vi "Audio Test.vi"(11 "Module Config":T9={"Name"="Base Station RF Test", "Parent Q"=refnum, "Is Child?"=FALSE, "Index"=0, "Dirs"={"Root"=path "", "Config"=path "C:/ATE/Config", "Logs"=path "C:/ATE/Logs", "Reports"=path "C:/ATE/Reports", "App Data"=path "C:/ProgramData/MAIN"}, "Simulate"=FALSE, "SimCtrl"=refnum}) -> ()   [LabVIEW 2018]
uses:
  <vilib>/KATE/Module/Module Config.ctl
  <vilib>/KATE/Queues/Q.Element.ctl
  <vilib>/KATE/Module/Module.Working Dirs.ctl
  Common/Utils/Results/Result.Measurement Item.ctl
  Common/Utils/Results/Result.Measurement and Attribute Item Status.ctl
  Common/Utils/Results/Result.Results Table Record.ctl
  Common/Utils/Results/Result XML/TestResult.SW Item.ctl
  <vilib>/KATE/Event Log/Event Notification/Event Log.Log Level.ctl
  TypeDefs/SoundCheck Config.ctl
  <vilib>/Utility/miscctls.llb/LVRectTypeDef.ctl
  <vilib>/KATE/Module/Module.SW Version Info.ctl
  <vilib>/KATE/Module/Window/Window.Task, Action.ctl
  Common/Utils/Functions/FunctDataMgr/FunctDataMgr.lvclass
  <vilib>/KATE/SeqMgr/SeqMgr.Result Info.ctl
  <vilib>/KATE/SeqMgr/SeqMgr.Result State Enum.ctl
  <vilib>/KATE/TCP-IP/Mgr/TCP-IP Mgr.Config.ctl
  Common/Utils/Errors/Error.Error Code List.ctl
  Common/Utils/TestExec/TestExec.WorkingDir.ctl
  Common/Utils/TestExec/TestExec.Test Start Message to Sta.ctl
  <vilib>/KATE/Event Log/Event Notification/Event Log.Notification Type.ctl
  Common/Utils/Results/Result.Attribute.ctl
  Common/Utils/Results/Result.Numeric.ctl
  Common/Utils/Results/Result.Limit Type.ctl
  Common/Utils/TestExec/TestExec.Health State Command.ctl
  <vilib>/Utility/config.llb/Read Key (Path).vi
  <vilib>/Utility/config.llb/Read Key (String).vi
  <vilib>/Utility/config.llb/Write Key (Path).vi
  <vilib>/Utility/config.llb/Write Key (String).vi
  <vilib>/KATE/Config/Stored Controls/Class.SaveCtrls.lvclass
  <vilib>/KATE/Queues/Queue Utils.lvlib
  <vilib>/KATE/Module/Module Utils.lvlib
  <vilib>/KATE/Event Log/Event Log.lvlib
  <vilib>/KATE/Scheduler/Scheduler.lvlib
  <vilib>/KATE/Menu/Menu Utils.lvlib
  <vilib>/KATE/Status/Status Utils.lvlib
  <vilib>/KATE/Event Log/Event Notification/Event Notification.lvclass
  <vilib>/KATE/TCP-IP/TCP-IP.lvlib
  <vilib>/KATE/Files/File Utils.lvlib
  <vilib>/KATE/SeqMgr/SeqMgr.lvlib
  <vilib>/KATE/Config/App Data/Class.AppData.lvclass
  <vilib>/KATE/Time/Time Utils.lvlib
  <vilib>/Utility/config.llb/NI_LVConfig.lvlib
panel:
  in  "Main Tab":enum32{"Operate", "Maint"}(tab)
  out "TE":bool
  out "Simulate Indication":string="Simulating Instruments"
  in  "Control Tab":enum32{"Test Control", "Misc Config"}(tab)
  in  "Parse Mic. Seal Results":bool
  in  "Parse Results":bool
  out "Enumerated":bool
  in  "Audio Seq Name":u16(ring)
  in  "Check UUT Enum Status":bool
  in  "Timeout(s)":dbl=500.0 caption="Time Out(s)" format="%.2f"
  in  "Get Top SN":bool
  in  "Mode":string="Production"
  in  "Run SoundCheck Script":bool
  in  "Archive Results":bool
  in  "Init UUT Folder":bool
  out "Start Time":timestamp
  in  "SN":string="ABC123"
  in  "Clear Errors":bool
  in  "Test Reset":bool
  out "Duration(s)":dbl format="%.2g"
  out "Status":string
  in  "Abort":bool
  in  "Result Data Tab":T1(tab)
  in  "Open Summary Dir":bool
  in  "UUT Dir":path caption="UUT Folder"
  in  "Open UUT Dir":bool
  in  "Open Archive Dir":bool
  in  "Filter":string
  in  "Show Only Failures":bool
  in  "Auto Scroll":bool=TRUE
  out "Results Table":T2[](array[typedef]) caption="Results"
  out "Graph Def File":path
  in  "SoundCheck Config":T3={"SeqDir"=path "C:/MTE/Audio Test/Config/SoundCheck/Sequences", "SoundCheckApp"=path "C:/SoundCheck 16.2-x64/SoundCheck 16.2 (x64).exe", "IP"="localhost", "Port"=4444, "Process Name"="SoundCheck 16.2 (x64)", "DataDir"=path "C:/MTE/Audio Test/Data/SoundCheck", "Window"=enum."Minimized"}
  out "Name Lookup":variant
  out "Name Lookup File":path
  in  "Undock HMD Util":bool
  in  "Undock Servo Util":bool
  out "Audio Utuil Dur(s)":dbl format="%.2f"
  out "AudUtil Running":bool
  in  "Run Audio Check":bool
  out "Audio Util Check":T4 {"Status" items=["LOG", "PASS", "FAIL", "ERROR"]}
  in  "Raw Results Tab":enum32{"Raw Result Data", "Other Data"}(tab)
  out "Measurement Data":T4[](array[typedef]) {"Status" items=["LOG", "PASS", "FAIL", "ERROR"]}
  out "Variables":string[][](array[string])
  out "UUT Properties":string[][](array[string])
  out "SW Items":T6[](array[typedef])
  out "Test Running":bool
  out "Error":errorcluster
  out "Ran to completion":bool
  in  "Both Mics":bool
  in  "Right Mic Cover":bool
  in  "Left Mic Cover":bool
  in  "Config - Reset":bool
  in  "Set Window Bounds":bool
  out "Temp Data Dir":path
  out "Archive Summary Dir":path
  out "Archive Dir":path
  in  "Logging Level":T7
  out "Old Window Bounds":T8={"Left"=2142, "Top"=133, "Right"=3354, "Bottom"=889}
  in  "New Window Bounds":T8={"Left"=212, "Top"=78, "Right"=1444, "Bottom"=899}
  out "Rev":string="v1.0.0"
  out "Error Status":string
  out "Title":string
  in  "Leave Maint":bool
  # "Cleanup:"
  # "Step                          Name                                                      Value                                    Units      LimType       LL           UL            Result          Code                     Description"
  # "Name                   PN                      Version                                        Notes"
  # "Name                                                       Value"
  # "Name                                                       Value"
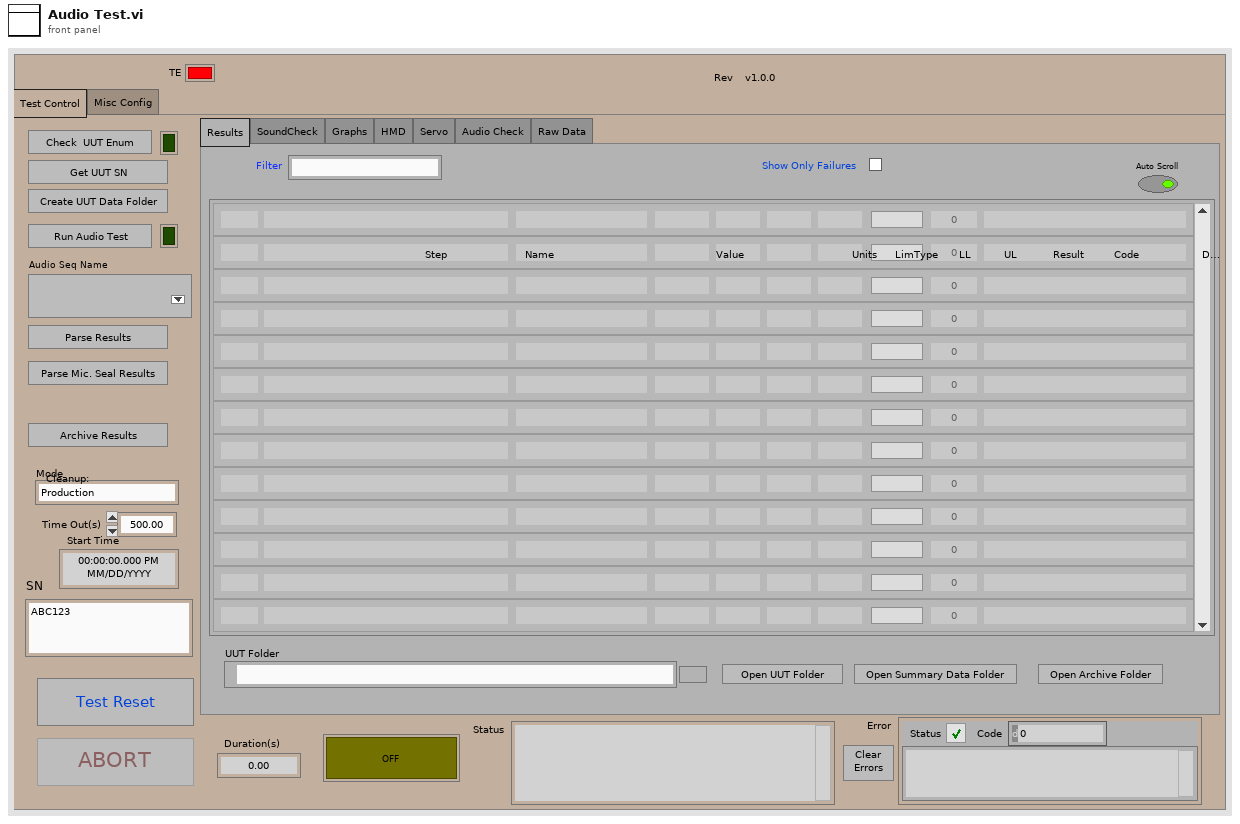
[diagram p1: front panel]
types:
  T1 = enum32{"Results", "SoundCheck", "Graphs", "HMD", "Servo", "Audio Check", "Raw Data"}
  T2 = typedef "Result.Results Table Record.ctl" = cluster{"Cnt":i32, "Step":string, "Category":string, "Name":string, "Value":string, "Units":string, "LimType":string, "LL":string, "UL":string, "Status":string, "Status Color":u32, "Code":i32, "Desc":string}
  T3 = typedef "SoundCheck Config.ctl" = cluster{"SeqDir":path, "SoundCheckApp":path, "IP":string, "Port":u16, "Process Name":string, "DataDir":path, "Window":enum16{"Normal", "Minimized", "Hidden"}}
  T4 = typedef "Result.Measurement Item.ctl" = cluster{"Cnt":i32, "Step":string, "Category":string, "Name":string, "Value":string, "Units":string, "LimType":string, "LL":string, "UL":string, "Status":T5, "Code":i32, "Desc":string, "Time":timestamp}
  T5 = typedef "Result.Measurement and Attribute Item Status.ctl" = i32
  T6 = typedef "TestResult.SW Item.ctl" = cluster{"Name":string, "PN":string, "Version":string, "Note":string}
  T7 = typedef "KATE_Lib.lvlib/Event Log.lvlib/Event Log.Log Level.ctl" = enum16{"Normal", "Verbose", "Debug0", "Debug1", "Debug2"}
  T8 = typedef "LVRectTypeDef.ctl" = cluster{"Left":i16, "Top":i16, "Right":i16, "Bottom":i16}
  T9 = typedef "KATE_Lib.lvlib/Module Utils.lvlib/Module Config.ctl" = cluster{"Name":string, "Parent Q":refnum<queue>, "Is Child?":bool, "Index":i32, "Dirs":T10, "Simulate":bool, "SimCtrl":refnum<vi>}
  T10 = typedef "KATE_Lib.lvlib/Module Utils.lvlib/Module.Working Dirs.ctl" = cluster{"Root":path, "Config":path, "Logs":path, "Reports":path, "App Data":path}
  T11 = typedef "KATE_Lib.lvlib/Module Utils.lvlib/Module.SW Version Info.ctl" = cluster{"AppName":string, "Company":string, "Version":string, "Description":string, "PN":string}
  T12 = typedef "KATE_Lib.lvlib/Module Utils.lvlib/Module Sys Info.ctl" = cluster{"Main Q":refnum<queue>, "Exe":bool, "SW Rev":T11, "Self Ref":refnum<vi>, "Main Tab":refnum<vi>, "Pane":refnum<vi>, "Stop":cluster{"Ref":refnum<event-registration>, "Event":refnum<user-event>}, "Cfg":T9, "Services":cluster{"Name":string, "vi ref":refnum<vi>}[], "Menu Ref":refnum<k9>, "CtrlStates":refnum<class "Class.SaveCtrls.lvclass">, "Docs":cluster{"Tags":string[], "Paths":path[]}, "Log":refnum<class "Event Notification.lvclass">, "Test Controls":refnum<vi>[], "Child Modules":cluster{"Name":string, "vi ref":refnum<vi>}[], "SW Items":string[][], "AppData":refnum<class "Class.AppData.lvclass">, "Subscriptions":refnum<class "Subscription.lvclass">}
  T13 = enum32{"Invalid", "Standard", "Closed", "Hidden", "Minimized", "Maximized"}
  T14 = typedef "KATE_Lib.lvlib/TCP-IP.lvlib/TCP-IP Mgr.Config.ctl" = cluster{"IP":string, "Port":u16, "Listener":bool, "Enable":bool}
  T15 = enum8{"Enabled", "Disabled", "Disabled and Grayed Out"}
  T16 = typedef "KATE_Lib.lvlib/Module Utils.lvlib/Window.Task, Action.ctl" = enum16{"Resize()", "Show Panel(Bool)", "Show Scroll Bars(Bool)", "Dock to SubPanel(SubPanel Ref)", "Undock from SubPanel()", "Return to SubPanel()", "Go To Maint Tab()", "Show Maint Tab(Bool)", "Open Block Diagram()"}
  T17 = typedef "TestExec.WorkingDir.ctl" = cluster{"Name":string, "Path":path}
  T18 = typedef "TestExec.Test Start Message to Sta.ctl" = cluster{"Test Name":string, "Start Time":timestamp, "UUT SN":string}
  T19 = typedef "KATE_Lib.lvlib/Event Log.lvlib/Event Log.Notification Type.ctl" = enum16{"Normal", "Warning", "Error", "Success"}
  T20 = cluster{"State":u16, "Norm":dbl[], "Covered":dbl[]}
  T21 = typedef "Result.Attribute.ctl" = cluster{"Cnt":i32, "Step":string, "Category":string, "Name":string, "Value":string, "Status":T5, "Code":i32, "Desc":string, "Time":timestamp}
  T22 = typedef "Result.Numeric.ctl" = cluster{"Cnt":i32, "Step":string, "Category":string, "Name":string, "Value":dbl, "Units":string, "LimType":T23, "LL":dbl, "UL":dbl, "Status":T5, "Code":i32, "Desc":string, "Time":timestamp}
  T23 = typedef "Result.Limit Type.ctl" = enum16{"None", "EQ", "NE", "GT", "LT", "GE", "LE", "GTLT", "GELE", "GELT", "GTLE", "LTGT", "LEGE", "LEGT", "LTGE", "Contains", "NotContains"}
  T24 = typedef "TestExec.Health State Command.ctl" = enum16{"Update", "Clear All", "Clear Warnings", "Clear Errors", "Set Warning", "Set Error"}
  T25 = typedef "KATE_Lib.lvlib/SeqMgr.lvlib/SeqMgr.Result Info.ctl" = cluster{"State":T26, "Code":i32, "Description":string}
  T26 = typedef "KATE_Lib.lvlib/SeqMgr.lvlib/SeqMgr.Result State Enum.ctl" = enum16{"None", "Passing", "Failing", "PASS", "FAIL", "ABORT", "ERROR"}
  T27 = cluster{"Archive":path, "ArchiveSum":path, "Temp Data":path, "UUTDir":path}
  T28 = cluster{"Lnch":bool, "FunctData":refnum<class "FunctDataMgr.lvclass">, "Timeout(s)":dbl, "Dirs":cluster{"Archive":path, "ArchiveSum":path, "Temp Data":path, "UUTDir":path}, "SN_Time":string, "Remote Test":bool, "ResultState":T25, "StaVer":i32, "Mic":cluster{"State":u16, "Norm":dbl[], "Covered":dbl[]}, "Script":string}
  T29 = typedef "Error.Error Code List.ctl" = i32
  T30 = typedef "NI_LVConfig.lvlib/Config Data RefNum.ctl" = refnum<k1>
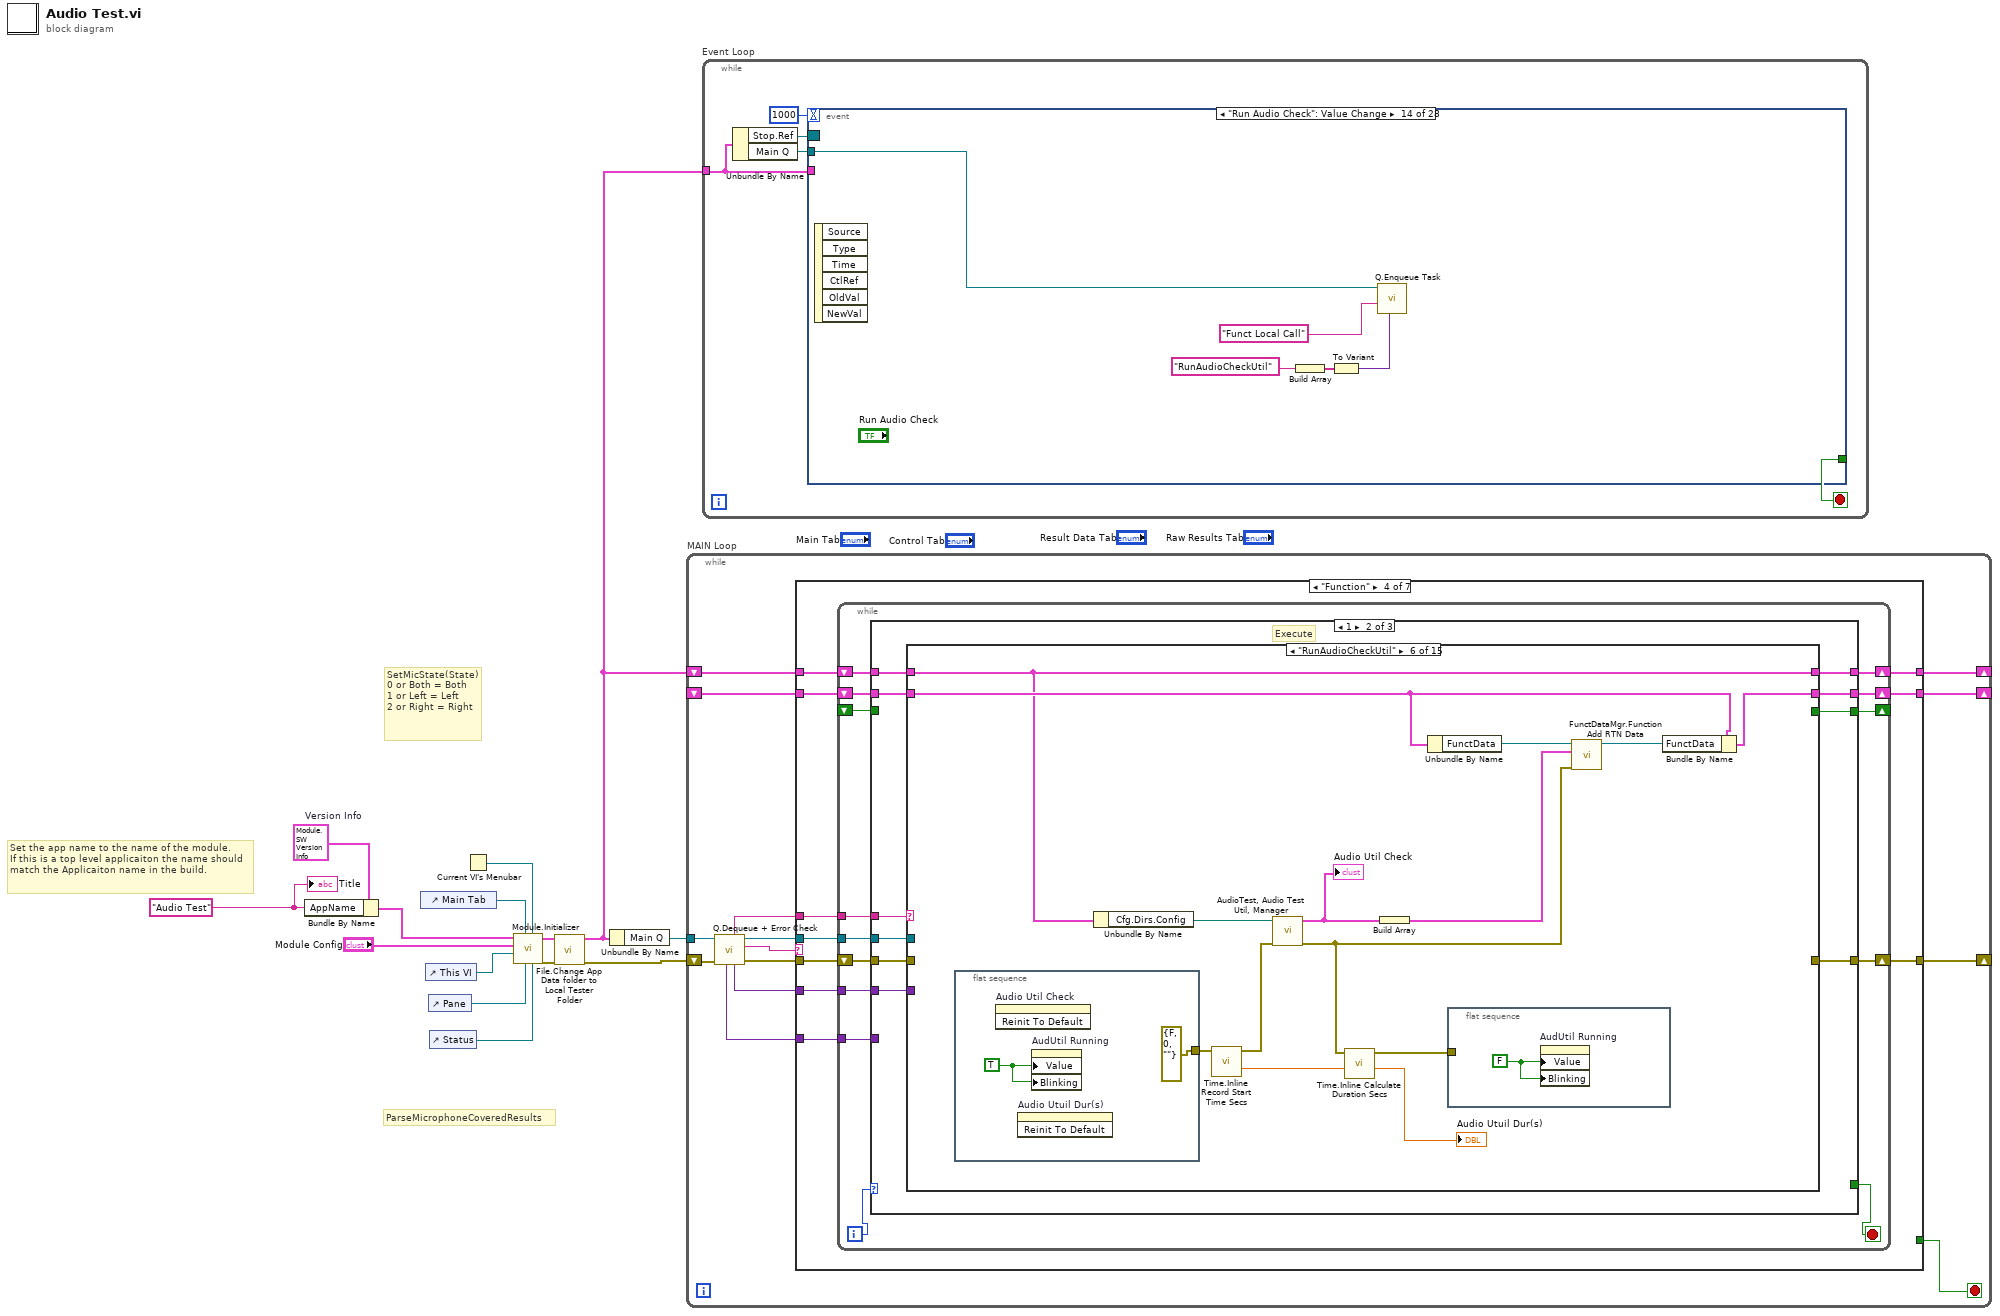
[diagram p0: block diagram]
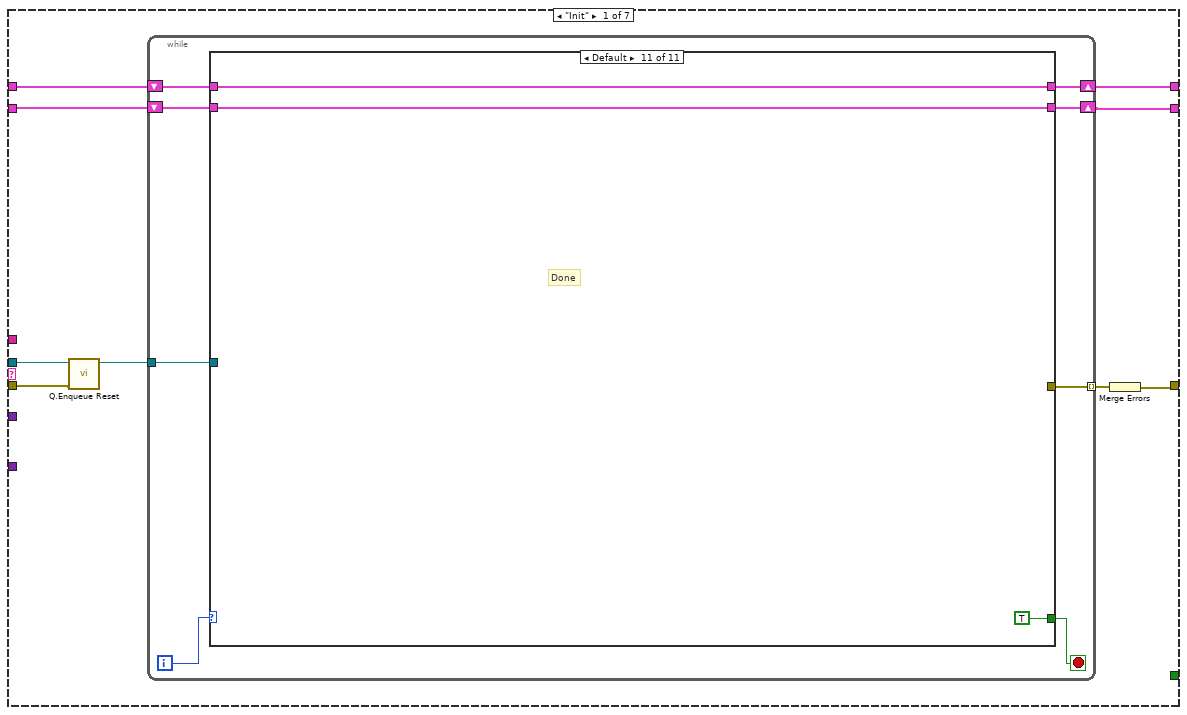
[diagram p2: hidden frame]
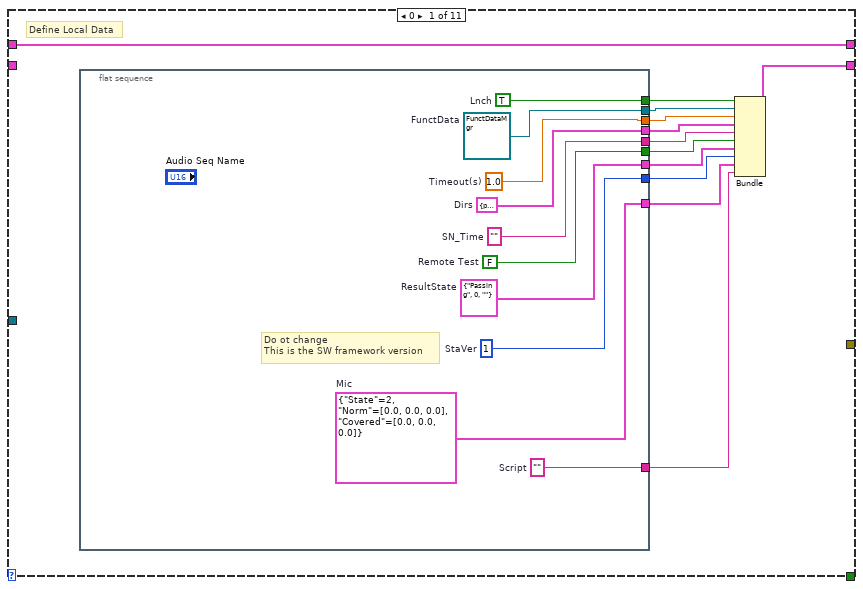
[diagram p3: hidden frame]
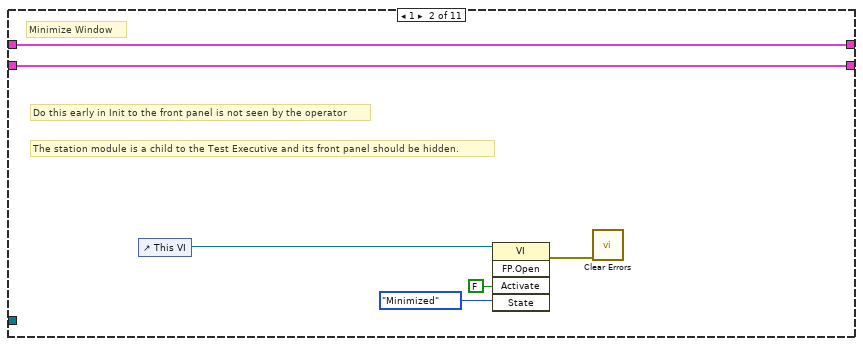
[diagram p4: hidden frame]
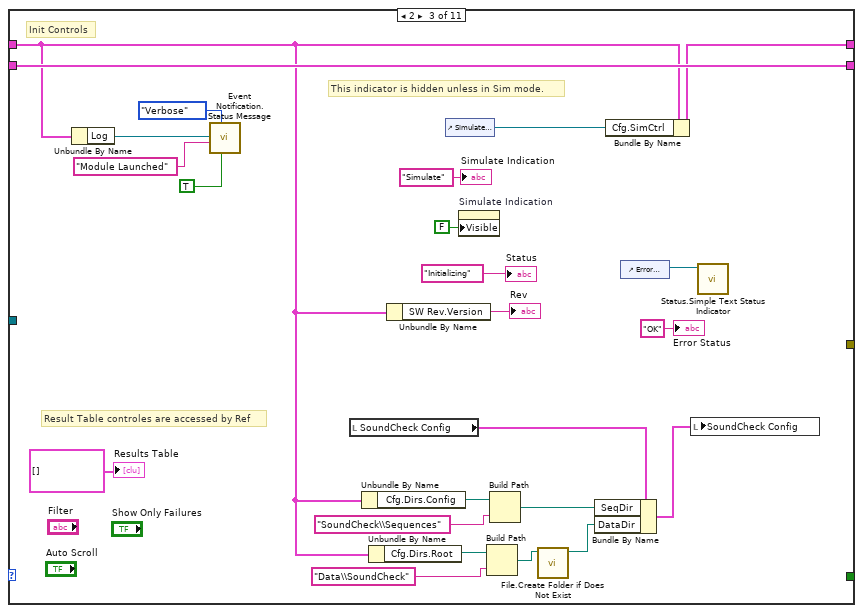
[diagram p5: hidden frame]
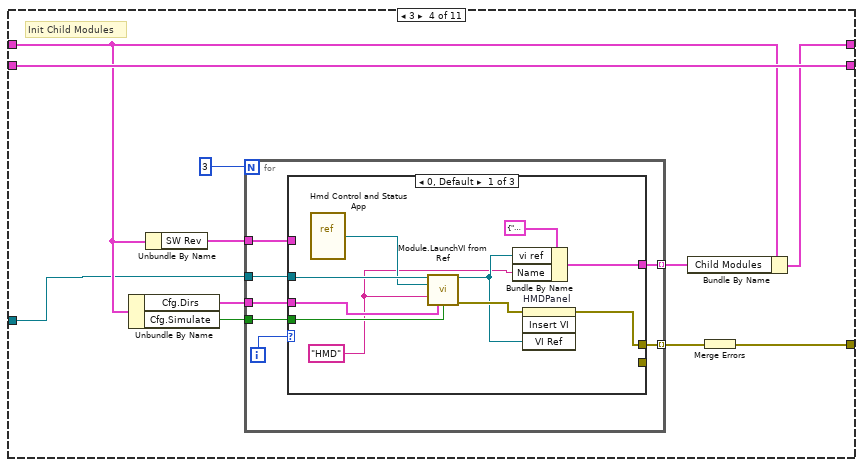
[diagram p6: hidden frame]
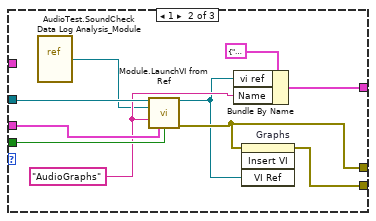
[diagram p7: hidden frame]
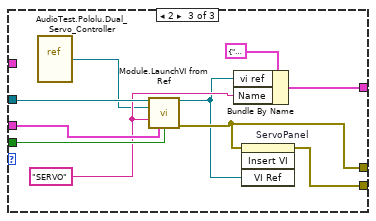
[diagram p8: hidden frame]
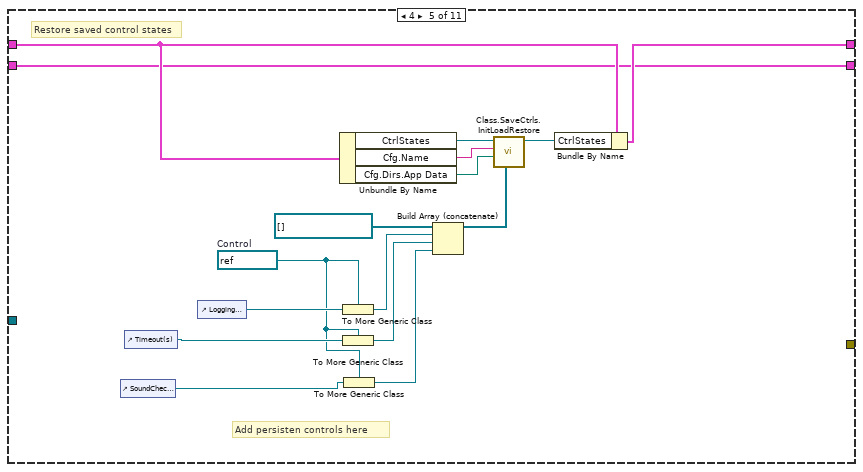
[diagram p9: hidden frame]
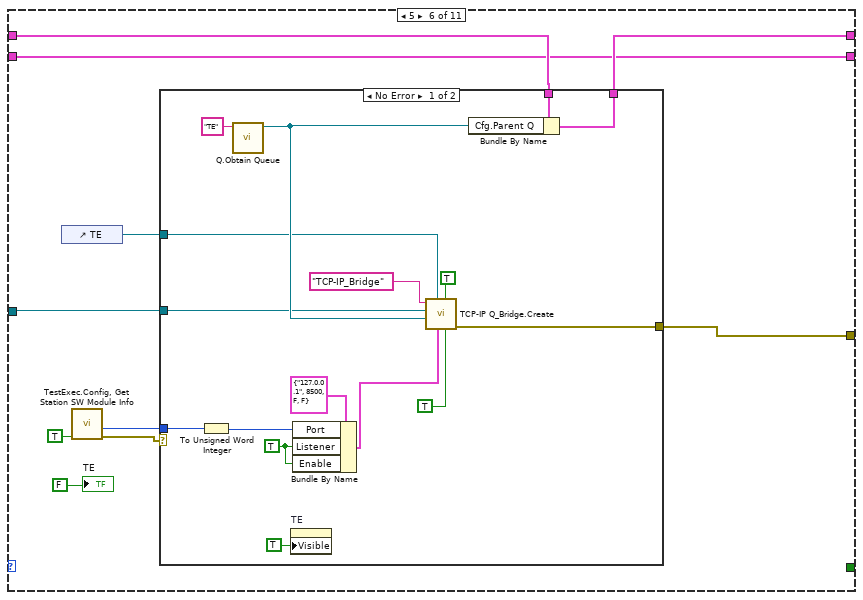
[diagram p10: hidden frame]
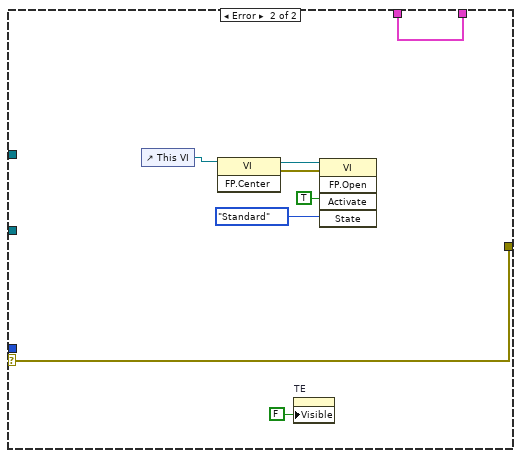
[diagram p11: hidden frame]
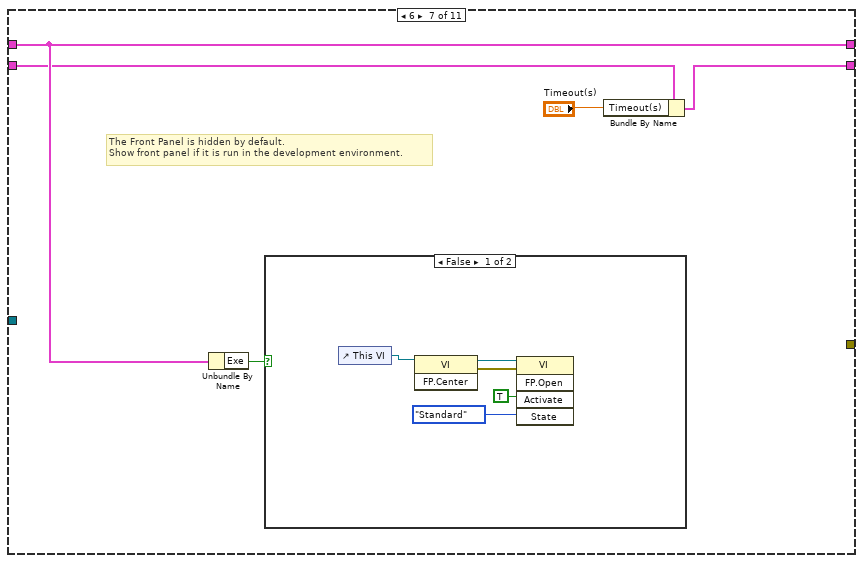
[diagram p12: hidden frame]
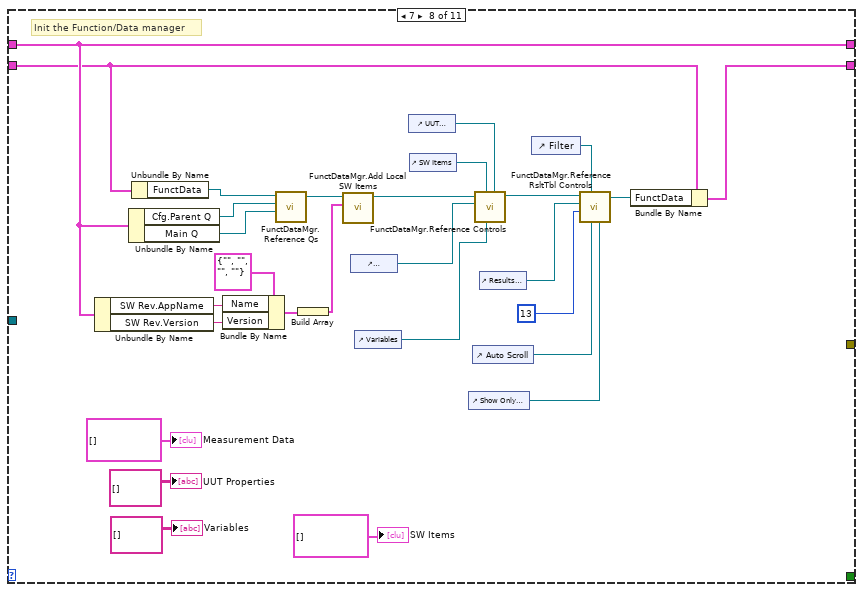
[diagram p14: hidden frame]
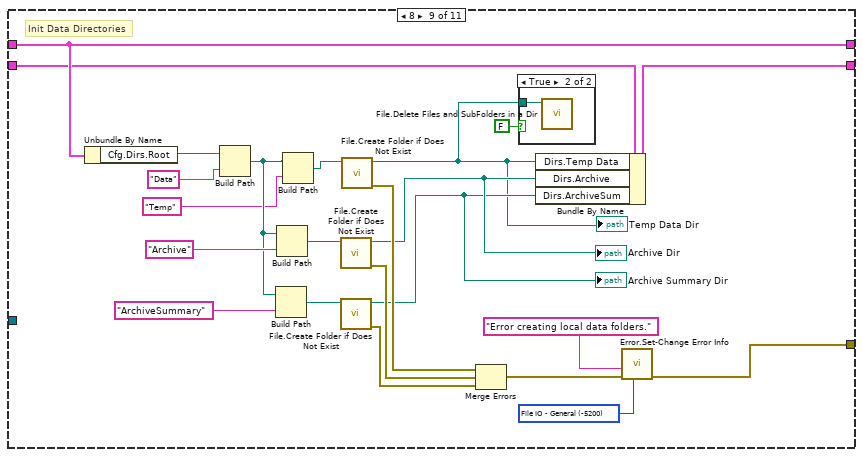
[diagram p15: hidden frame]
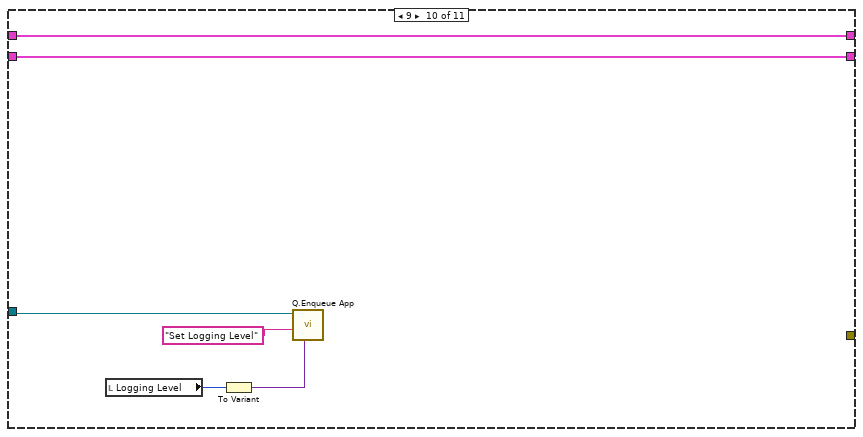
[diagram p17: hidden frame]
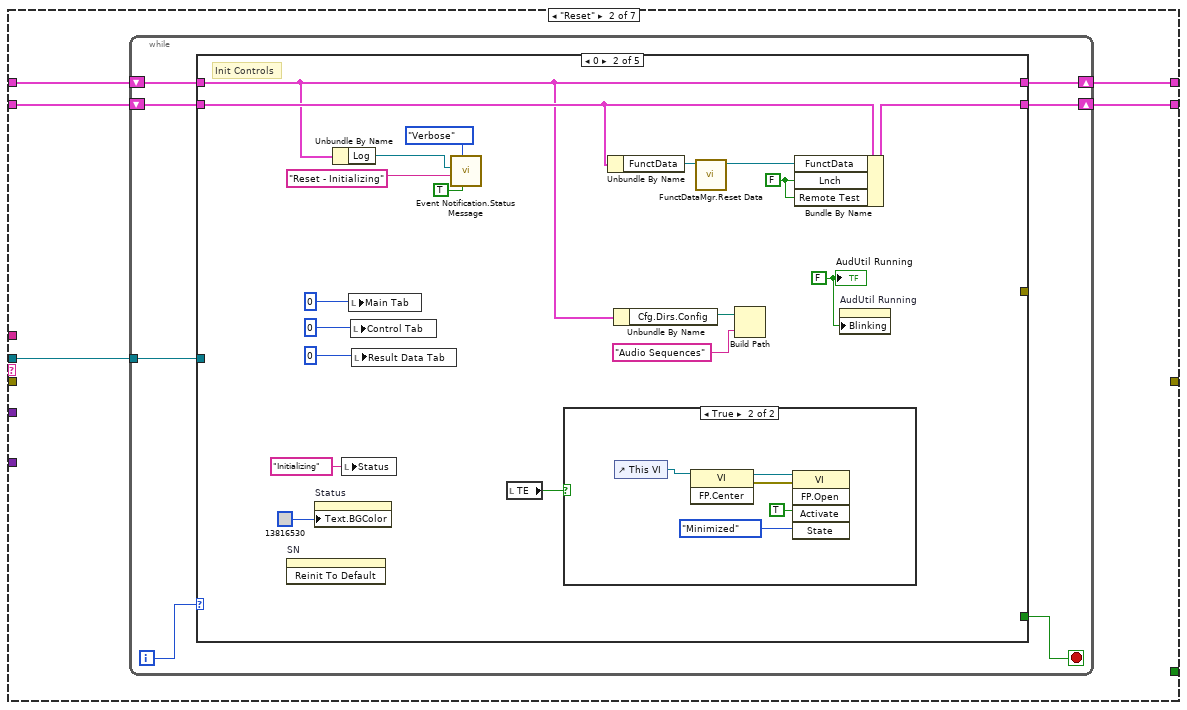
[diagram p18: hidden frame]
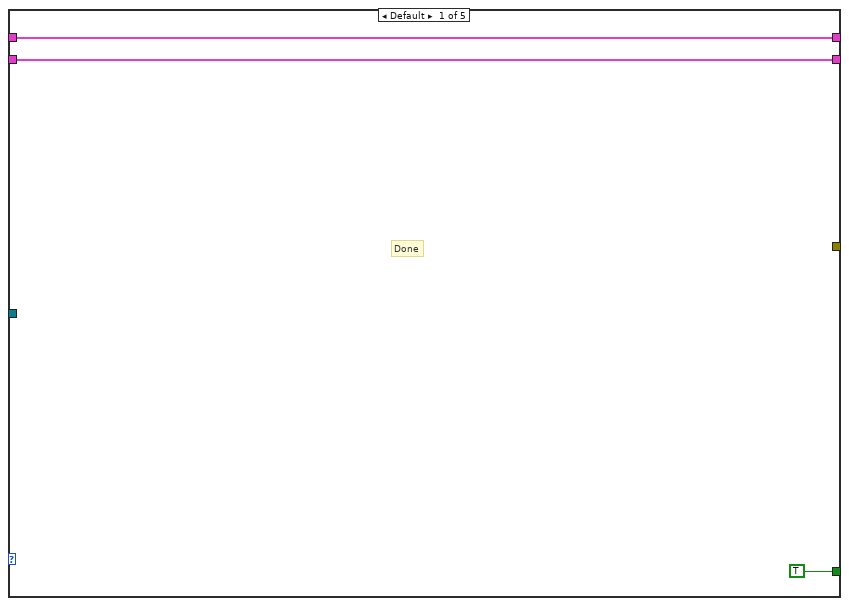
[diagram p19: hidden frame]
diagram:
  w8 = T11 {"AppName"="ModuleX", "Company"="CompanyX", "Version"="1.0", "Description"="This app is being developed.", "PN"=""}  # Version Info
  w5 = "Audio Test"
  # "ParseMicrophoneCoveredResults"
  # "SetMicState(State)\n0 or Both = Both\n1 or Left = Left\n2 or Right = Right"
  # "Set the app name to the name of the module.\nIf this is a top level applicaiton the name should match the Applicaiton name in the build."
  n1 = Bundle By Name(cluster=w8, "AppName"=w5) -> (w7:T11)
  n2 = control-ref of="Main Tab"() -> (w13:refnum<vi>)
  n3 = control-ref of="This VI"() -> (w12:refnum<vi>)
  n4 = control-ref of="Pane"() -> (w11:refnum<vi>)
  n5 = control-ref of="Status"() -> (w6:refnum<vi>)
  n6 = Current VI's Menubar() -> (w10:refnum<k9>)
  n7 = call <vilib>:"Module.Initializer.vi"("StatusTxtBx"=w6, "Menu Ref"=w10, "Pane"=w11, "Main Tab"=w13, "Self Ref"=w12, "Module Config"="Module Config", "SW Rev"=w7) -> ("error out"=w3:errorcluster, "Sys"=w2:T12)  [unwired: 3 in]
  n8 = call "File.Change App Data folder to Local Tester Folder.vi"("Sys"=w2) -> ("Sys Out"=w1:T12)  [unwired: 9 in, 1 out]
  n9 = Unbundle By Name(w1) -> ("Main Q"=w4:refnum<queue>)
  n10 = while "MAIN Loop" {
    shift-right: [w23] -> _
    shift-left: w3 -> [w21]
    shift-right: [w24] -> _
    shift-left: _ -> [w27]
    shift-right: [w25] -> _
    shift-left: w1 -> [w26]
    tunnel: w4 -> [w20]
    stop <- w16 stop-if-true
    n11 = call <vilib>:"Q.Dequeue + Error Check.vi"("Error In"=w21, "Q In"=w20) -> ("error out"=w22:errorcluster, "Cmd"=w15:string, "Q Out"=w19:refnum<queue>, "Data1"=w18:variant, "Sub"=w14:string, "Data2"=w17:variant)  [unwired: 4 in]
    n12 = case shown="\"Function\"" w15 {
      selector: w15 -> [_ _ _ _ _ w1245 _]
      tunnel: w27 -> [w32 w269 w368 w838 w1194 w1251 w1298]
      tunnel: w26 -> [w34 w270 w369 w839 w1195 w1250 w1294]
      tunnel: [w33 w268 w367 w837 w1193 w1250 w1295] -> w25
      tunnel: [w31 w267 w366 w836 w1192 w1249 w1298] -> w24
      tunnel: [w28 _ w360 w834 _ w1248 w1300] -> w23
      tunnel: w22 -> [w35 _ w362 w835 _ w1244 _]
      tunnel: w19 -> [w36 w266 w363 w832 w1198 w1247 _]
      tunnel: w18 -> [_ _ w364 w831 w1197 w1243 _]
      tunnel: w17 -> [_ _ w361 w830 w1196 _ _]
      tunnel: w14 -> [_ _ w365 w833 w1199 w1246 _]
      tunnel: [_ _ _ _ _ _ TRUE] -> w16
      frame "Init" {
        n13 = call <vilib>:"Q.Enqueue Reset.vi"("Error In"=w35, "Q In"=w36) -> ("Q Out"=w30:refnum<queue>)  [unwired: 8 in, 1 out]
        n14 = while {
          shift-right: [w43] -> w33
          shift-left: w34 -> [w44]
          shift-right: [w41] -> w31
          shift-left: w32 -> [w42]
          tunnel: w30 -> [w39]
          tunnel: [w38] -> w29 mode=indexing
          i -> [w37]
          stop <- w40 stop-if-true
          n15 = case shown="Default" w37 {
            tunnel: w44 -> [w56 w72 w77 w99 w151 w164 w198 w214 w255 w262 w265]
            tunnel: [w56 w72 w87 w100 w149 w163 w198 w214 w255 w262 w265] -> w43
            tunnel: w42 -> [_ w69 w96 w107 w148 w162 w197 w211 w254 w261 w264]
            tunnel: [w55 w69 w96 w107 w148 w162 w196 w212 w253 w261 w264] -> w41
            tunnel: [_ _ _ _ _ _ _ _ _ _ TRUE] -> w40
            tunnel: w39 -> [_ _ _ w98 _ w165 _ _ _ w258 _]
            tunnel: [_ _ _ w101 _ w161 _ _ w243 _ _] -> w38
            frame 0 {
              # "Define Local Data"
              n16 = flat-sequence {
                tunnel: [w66] -> w54
                tunnel: [w65] -> w53
                tunnel: [w64] -> w52
                tunnel: [w63] -> w51
                tunnel: [w62] -> w50
                tunnel: [w61] -> w49
                tunnel: [w60] -> w48
                tunnel: [w59] -> w47
                tunnel: [w58] -> w46
                tunnel: [w57] -> w45
                frame #0 {
                  w57 = ""  # Script
                  w58 = T20 {"State"=2, "Norm"=[0.0, 0.0, 0.0], "Covered"=[0.0, 0.0, 0.0]}  # Mic
                  w59 = 1  # StaVer
                  w60 = T25 {"State"=enum."Passing", "Code"=0, "Description"=""}  # ResultState
                  w61 = FALSE  # Remote Test
                  w62 = ""  # SN_Time
                  w65 = refnum<class "FunctDataMgr.lvclass"> refnum  # FunctData
                  w63 = T27 {"Archive"=path "", "ArchiveSum"=path "", "Temp Data"=path "", "UUTDir"=path ""}  # Dirs
                  w64 = 1.0  # Timeout(s)
                  w66 = TRUE  # Lnch
                  # "Do ot change\nThis is the SW framework version"
                }
              }
              n17 = Bundle("Lnch"=w54, "FunctData"=w53, "Timeout(s)"=w52, "Dirs"=w51, "SN_Time"=w50, "Remote Test"=w49, "ResultState"=w48, "StaVer"=w47, "Mic"=w46, "Script"=w45) -> (w55:T28)  [unwired: 1 in]
            }
            frame 1 {
              # "The station module is a child to the Test Executive and its front panel should be hidden."
              # "Do this early in Init to the front panel is not seen by the operator"
              # "Minimize Window"
              n18 = control-ref of="This VI"() -> (w68:refnum<vi>)
              n19 = invoke class="VI" method="FP.Open"(reference=w68, "Activate"=FALSE ("Activate?"), "State"=T13."Minimized") -> (error out=w67:errorcluster)  [unwired: 2 in, 4 out]
              n20 = call <vilib>:"Clear Errors.vi"("error in (no error)"=w67) -> ()  [unwired: 5 in, 2 out]
            }
            frame 2 {
              # "Init Controls"
              # "This indicator is hidden unless in Sim mode."
              # "Result Table controles are accessed by Ref"
              n21 = Unbundle By Name(w77) -> ("Log"=w94:refnum<class "Event Notification.lvclass">)
              n22 = call <vilib>:"Event Notification.Status Message.vi"("Log"=TRUE, "Level"=Event_Log.Log_Level."Verbose", "Message"="Module Launched", "Event Notification in"=w94) -> ()  [unwired: 8 in]
              n23 = local read "SoundCheck Config"() -> (w82:T3)
              n24 = Unbundle By Name(w77) -> ("Cfg.Dirs.Config"=w80:path)
              n25 = Unbundle By Name(w77) -> ("Cfg.Dirs.Root"=w76:path)
              n26 = Unbundle By Name(w77) -> ("SW Rev.Version"=→"Rev":string)
              n27 = control-ref of="Simulate Indication"() -> (w88:refnum<vi>)
              n28 = property on="Simulate Indication" class="Str"("Visible"=FALSE) -> ()  [unwired: 2 in, 2 out]
              n29 = Build Path(base path=w76, name or relative path="Data\\SoundCheck") -> (appended path=w73:path)
              n30 = Build Path(base path=w80, name or relative path="SoundCheck\\Sequences") -> (appended path=w78:path)
              n31 = call <vilib>:"File.Create Folder if Does Not Exist.vi"("Path"=w73) -> ("Dup Path"=w74:path)  [unwired: 8 in, 2 out]
              n32 = Bundle By Name(cluster=w82, "SeqDir"=w78, "DataDir"=w74) -> (w81:T3)
              n33 = Bundle By Name(cluster=w77, "Cfg.SimCtrl"=w88) -> (w87:T12)
              n34 = control-ref of="Error Status"() -> (w86:refnum<vi>)
              n35 = local write "SoundCheck Config"(w81) -> ()
              n36 = call <vilib>:"Status.Simple Text Status Indicator.vi"("Status TextBox"=w86) -> ()  [unwired: 10 in, 1 out]
              "Results Table" <- T2[] [] ("Results Table")
              "Simulate Indication" <- "Simulate" ("Simulate Indication")
              "Status" <- "Initializing" ("Status")
              "Error Status" <- "OK" ("Error Status")
            }
            frame 3 {
              # "Init Child Modules"
              n37 = Unbundle By Name(w99) -> ("Cfg.Dirs"=w104:T10, "Cfg.Simulate"=w105:bool)
              n38 = Unbundle By Name(w99) -> ("SW Rev"=w103:T11)
              n39 = for {
                N: 3 -> [_]
                tunnel: w103 -> [w114]
                tunnel: [w109] -> w97 mode=indexing
                tunnel: w98 -> [w112]
                tunnel: w104 -> [w111]
                tunnel: w105 -> [w110]
                tunnel: [w108] -> w106 mode=indexing
                i -> [w113]
                n40 = case shown="0, Default" w113 {
                  tunnel: w114 -> [_ _ _]
                  tunnel: w112 -> [w124 w134 w144]
                  tunnel: w111 -> [w118 w132 w142]
                  tunnel: w110 -> [w117 w131 w141]
                  tunnel: [w122 w133 w143] -> w109
                  tunnel: [w121 w128 w138] -> w108
                  tunnel: [_ w127 w137] -> _
                  frame 0, Default {
                    w115 = "HMD"
                    n41 = vi-ref "Hmd Control and Status App.vi"() -> (w123:refnum<vi>)
                    n42 = call <vilib>:"Module.LaunchVI from Ref.vi"("Parent Q"=w124, "VI Ref In"=w123, "Q Name"=w115, "Working Dirs"=w118, "Simulate"=w117) -> ("VI Ref Out"=w119:refnum<vi>, "error out"=w120:errorcluster)  [unwired: 8 in, 1 out]
                    n43 = Bundle By Name(cluster=cluster{"Name":string, "vi ref":refnum<vi>} {"Name"="", "vi ref"=refnum} ("Service"), "vi ref"=w119, "Name"=w115) -> (w122:cluster{"Name":string, "vi ref":refnum<vi>})
                    n44 = invoke on="HMDPanel" class="SubPnl" method="Insert VI"(error in=w120, "VI Ref"=w119) -> (error out=w121:errorcluster)  [unwired: 2 in, 3 out]
                  }
                  frame 1 {
                    w129 = "AudioGraphs"
                    n45 = vi-ref "AudioTest.SoundCheck Data Log Analysis_Module.vi"() -> (w125:refnum<vi>)
                    n46 = call <vilib>:"Module.LaunchVI from Ref.vi"("Parent Q"=w134, "VI Ref In"=w125, "Q Name"=w129, "Working Dirs"=w132, "Simulate"=w131) -> ("VI Ref Out"=w126:refnum<vi>, "error out"=w128:errorcluster)  [unwired: 8 in, 1 out]
                    n47 = Bundle By Name(cluster=cluster{"Name":string, "vi ref":refnum<vi>} {"Name"="", "vi ref"=refnum} ("Service"), "vi ref"=w126, "Name"=w129) -> (w133:cluster{"Name":string, "vi ref":refnum<vi>})
                    n48 = invoke on="Graphs" class="SubPnl" method="Insert VI"(error in=w128, "VI Ref"=w126) -> (error out=w127:errorcluster)  [unwired: 2 in, 3 out]
                  }
                  frame 2 {
                    w139 = "SERVO"
                    n49 = vi-ref "AudioTest.Pololu.Dual_Servo_Controller.vi"() -> (w135:refnum<vi>)
                    n50 = call <vilib>:"Module.LaunchVI from Ref.vi"("Parent Q"=w144, "VI Ref In"=w135, "Q Name"=w139, "Working Dirs"=w142, "Simulate"=w141) -> ("VI Ref Out"=w136:refnum<vi>, "error out"=w138:errorcluster)  [unwired: 8 in, 1 out]
                    n51 = Bundle By Name(cluster=cluster{"Name":string, "vi ref":refnum<vi>} {"Name"="", "vi ref"=refnum} ("Service"), "vi ref"=w136, "Name"=w139) -> (w143:cluster{"Name":string, "vi ref":refnum<vi>})
                    n52 = invoke on="ServoPanel" class="SubPnl" method="Insert VI"(error in=w138, "VI Ref"=w136) -> (error out=w137:errorcluster)  [unwired: 2 in, 3 out]
                  }
                }
              }
              n53 = Bundle By Name(cluster=w99, "Child Modules"=w97) -> (w100:T12)
              n54 = Merge Errors(w106) -> (w101:errorcluster)
            }
            frame 4 {
              w146 = refnum<vi> refnum  # Control
              # "Add persisten controls here"
              # "Restore saved control states"
              n55 = control-ref of="SoundCheck Config"() -> (w147:refnum<vi>)
              n56 = control-ref of="Timeout(s)"() -> (w150:refnum<vi>)
              n57 = control-ref of="Logging Level"() -> (w160:refnum<vi>)
              n58 = Unbundle By Name(w151) -> ("CtrlStates"=w156:refnum<class "Class.SaveCtrls.lvclass">, "Cfg.Name"=w154:string, "Cfg.Dirs.App Data"=w155:path)
              n59 = To More Generic Class(target class=w146, reference=w160) -> (generic class reference=w158:refnum<vi>)
              n60 = To More Generic Class(target class=w146, reference=w150) -> (generic class reference=w159:refnum<vi>)
              n61 = To More Generic Class(target class=w146, reference=w147) -> (generic class reference=w145:refnum<vi>)
              n62 = Build Array (concatenate)(refnum<vi>[] [], w158, w159, w145) -> (w157:refnum<vi>[])
              n63 = call-dynamic "Class.SaveCtrls.InitLoadRestore.vi"("Ctrl Array"=w157, "Module Data Dir"=w155, "Module Name"=w154, "CtrlStates In"=w156) -> ("CtrlStates"=w152:refnum<class "Class.SaveCtrls.lvclass">)  [unwired: 6 in, 1 out]
              n64 = Bundle By Name(cluster=w151, "CtrlStates"=w152) -> (w149:T12)
            }
            frame 5 {
              n65 = control-ref of="TE"() -> (w170:refnum<vi>)
              n66 = call "TestExec.Config, Get Station SW Module Info.vi"("Error if File Doesn't Exist"=TRUE) -> ("error out"=w169:errorcluster, "Station IP Port"=w168:i32)  [unwired: 7 in, 2 out]
              n67 = case shown="No Error" w169 {
                selector: w169 -> [_ w193]
                tunnel: w164 -> [w186 w194]
                tunnel: [w185 w194] -> w163
                tunnel: w168 -> [w178 _]
                tunnel: w165 -> [w175 _]
                tunnel: [w174 w193] -> w161
                tunnel: w170 -> [w173 _]
                frame No Error {
                  w179 = TRUE ("Listener")
                  n68 = To Unsigned Word Integer(number=w178) -> (unsigned 16bit integer=w177:u16)
                  n69 = call <vilib>:"Q.Obtain Queue.vi"("Q Name"="TE") -> ("Q Out"=w183:refnum<queue>)  [unwired: 8 in, 2 out]
                  n70 = property on="TE" class="Bool (strict)"("Visible"=TRUE) -> ()  [unwired: 2 in, 2 out]
                  n71 = Bundle By Name(cluster=T14 {"IP"="127.0.0.1", "Port"=8500, "Listener"=FALSE, "Enable"=FALSE} ("Config"), "Port"=w177, "Listener"=w179, "Enable"=w179) -> (w180:T14)
                  n72 = call <vilib>:"TCP-IP Q_Bridge.Create.vi"("Auto Exit"=TRUE, "Notification"=TRUE, "Config"=w180, "StatusCtrlRef"=w173, "Q_DataOut"=w183, "Q_DataIn"=w175, "Control Q Name"="TCP-IP_Bridge" ("Control Q")) -> ("Error Out"=w174:errorcluster)  [unwired: 3 in, 1 out]
                  n73 = Bundle By Name(cluster=w186, "Cfg.Parent Q"=w183) -> (w185:T12)
                }
                frame Error {
                  n74 = control-ref of="This VI"() -> (w189:refnum<vi>)
                  n75 = invoke class="VI" method="FP.Center"(reference=w189) -> (reference out=w190:refnum<vi>, error out=w191:errorcluster)  [unwired: 2 in, 1 out]
                  n76 = property on="TE" class="Bool (strict)"("Visible"=FALSE) -> ()  [unwired: 2 in, 2 out]
                  n77 = invoke class="VI" method="FP.Open"(reference=w190, error in=w191, "Activate"=TRUE ("Activate?"), "State"=T13."Standard") -> ()  [unwired: 1 in, 5 out]
                }
              }
              "TE" <- FALSE ("Sta")
            }
            frame 6 {
              # "The Front Panel is hidden by default.\nShow front panel if it is run in the development environment."
              n78 = Unbundle By Name(w198) -> ("Exe"=w199:bool)
              n79 = case shown="False" w199 {
                frame False {
                  n80 = control-ref of="This VI"() -> (w202:refnum<vi>)
                  n81 = invoke class="VI" method="FP.Center"(reference=w202) -> (reference out=w203:refnum<vi>, error out=w204:errorcluster)  [unwired: 2 in, 1 out]
                  n82 = invoke class="VI" method="FP.Open"(reference=w203, error in=w204, "Activate"=TRUE ("Activate?"), "State"=T13."Standard") -> ()  [unwired: 1 in, 5 out]
                }
                frame True {
                }
              }
              n83 = Bundle By Name(cluster=w197, "Timeout(s)"="Timeout(s)") -> (w196:T28)
            }
            frame 7 {
              # "Init the Function/Data manager"
              n84 = Unbundle By Name(w214) -> ("SW Rev.AppName"=w219:string, "SW Rev.Version"=w220:string)
              n85 = Unbundle By Name(w214) -> ("Cfg.Parent Q"=w222:refnum<queue>, "Main Q"=w223:refnum<queue>)
              n86 = Unbundle By Name(w211) -> ("FunctData"=w210:refnum<class "FunctDataMgr.lvclass">)
              n87 = Bundle By Name(cluster=T6 {"Name"="", "PN"="", "Version"="", "Note"=""} ("SW"), "Name"=w219, "Version"=w220) -> (w218:T6)
              n88 = call "FunctDataMgr.Reference Qs.vi"("Q Local"=w223, "Q Parent"=w222, "FunctDataMgr in"=w210) -> ("FunctDataMgr"=w224:refnum<class "FunctDataMgr.lvclass">)  [unwired: 7 in, 1 out]
              n89 = Build Array(w218) -> (w221:T6[])
              n90 = call "FunctDataMgr.Add Local SW Items.vi"("Local SW Items"=w221, "FunctDataMgr in"=w224) -> ("FunctDataMgr"=w225:refnum<class "FunctDataMgr.lvclass">)  [unwired: 8 in, 1 out]
              n91 = control-ref of="Measurement Data"() -> (w205:refnum<vi>)
              n92 = control-ref of="Variables"() -> (w232:refnum<vi>)
              n93 = control-ref of="UUT Properties"() -> (w226:refnum<vi>)
              n94 = control-ref of="SW Items"() -> (w227:refnum<vi>)
              n95 = control-ref of="Show Only Failures"() -> (w230:refnum<vi>)
              n96 = control-ref of="Auto Scroll"() -> (w231:refnum<vi>)
              n97 = call "FunctDataMgr.Reference Controls.vi"("UUTProps"=w226, "Vars"=w232, "SWItems"=w227, "Ctrls.MeasData"=w205, "FunctDataMgr in"=w225) -> ("FunctDataMgr"=w217:refnum<class "FunctDataMgr.lvclass">)  [unwired: 5 in, 1 out]
              n98 = control-ref of="Results Table"() -> (w229:refnum<vi>)
              n99 = control-ref of="Filter"() -> (w228:refnum<vi>)
              n100 = call "FunctDataMgr.Reference RsltTbl Controls.vi"("ShowOnlyFail"=w230, "AutoScroll"=w231, "Filter"=w228, "Visible Rows"=13, "RsltTbl"=w229, "FunctDataMgr in"=w217) -> ("FunctDataMgr"=w213:refnum<class "FunctDataMgr.lvclass">)  [unwired: 4 in, 1 out]
              n101 = Bundle By Name(cluster=w211, "FunctData"=w213) -> (w212:T28)
              "Measurement Data" <- T4[] [] ("Numeric Data")
              "UUT Properties" <- string[][] [] ("UUT Properties")
              "Variables" <- string[][] [] ("Variables")
              "SW Items" <- T6[] [] ("SW Items")
            }
            frame 8 {
              w242 = T29 -5200 items=["No Error"=0, "Abort"=-2, "Misc"=-5000, "Fixture Error"=-5100, "File IO - General"=-5200, "FIle IO - Config Error"=-5201, "Instrument - General"=-5300, "Instrument - Serial Com"=-5301, "Instrument - Camera"=-5302, "Instrument - PS"=-5303, "Instrument - Oscilloscope"=-5304, "Instrument - Function Gen"=-5305, "Instrument - Load"=-5306, "Instrument - Meter"=-5307, "Instrument - Power Control"=-5308, "Instrument - Motion"=-5309, "Instrument - RF"=-5310, "System Exe"=-5400, "Image Processing"=-5500, "Communication"=-5600, "Script - Syntax Error"=-6000, "Script - Invalid Name or Param"=-6100, "Script - Timeout"=-6200, "Invalid Data"=-6300, "FW Update Error"=-6500] ("Std Code")
              # "Init Data Directories"
              n102 = Unbundle By Name(w255) -> ("Cfg.Dirs.Root"=w252:path)
              n103 = Build Path(base path=w252, name or relative path="Data") -> (appended path=w240:path)
              n104 = Build Path(base path=w240, name or relative path="ArchiveSummary") -> (appended path=w237:path)
              n105 = Build Path(base path=w240, name or relative path="Archive") -> (appended path=w250:path)
              n106 = Build Path(base path=w240, name or relative path="Temp") -> (appended path=w239:path)
              n107 = call <vilib>:"File.Create Folder if Does Not Exist.vi"("Path"=w250) -> ("error out"=w246:errorcluster, "Dup Path"=w236:path)  [unwired: 8 in, 1 out]
              "Archive Dir" <- w236
              n108 = call <vilib>:"File.Create Folder if Does Not Exist.vi"("Path"=w237) -> ("error out"=w245:errorcluster, "Dup Path"=w235:path)  [unwired: 8 in, 1 out]
              "Archive Summary Dir" <- w235
              n109 = call <vilib>:"File.Create Folder if Does Not Exist.vi"("Path"=w239) -> ("error out"=w247:errorcluster, "Dup Path"=w233:path)  [unwired: 8 in, 1 out]
              "Temp Data Dir" <- w233
              n110 = Merge Errors(w247, w246, w245) -> (w244:errorcluster)
              n111 = case shown="True" FALSE {
                tunnel: w233 -> [_ w256]
                frame False {
                }
                frame True {
                  n112 = call <vilib>:"File.Delete Files and SubFolders in a Dir.vi"("Dir"=w256) -> ()  [unwired: 9 in, 2 out]
                }
              }
              n113 = Bundle By Name(cluster=w254, "Dirs.Temp Data"=w233, "Dirs.Archive"=w236, "Dirs.ArchiveSum"=w235) -> (w253:T28)
              n114 = call "Error.Set-Change Error Info.vi"("Std Code"=w242, "error in"=w244, "Description"="Error creating local data folders.") -> ("error out"=w243:errorcluster)  [unwired: 8 in]
            }
            frame 9 {
              n115 = local read "Logging Level"() -> (w257:T7)
              n116 = To Variant(anything=w257) -> (Variant=w259:variant)
              n117 = call <vilib>:"Q.Enqueue App.vi"("Data1"=w259, "Task Name"="Set Logging Level", "Q In"=w258) -> ()  [unwired: 7 in, 2 out]
            }
            frame Default {
              # "Done"
            }
          }
        }
        n118 = Merge Errors(w29) -> (w28:errorcluster)
      }
      frame "Reset" {
        n119 = while {
          shift-right: [w275] -> w268
          shift-left: w270 -> [w276]
          shift-right: [w273] -> w267
          shift-left: w269 -> [w274]
          tunnel: w266 -> [w271]
          i -> [w277]
          stop <- w272 stop-if-true
          n120 = case shown="0" w277 {
            tunnel: w276 -> [w279 w285 w307 w352 w358]
            tunnel: [w279 w285 w307 w352 w358] -> w275
            tunnel: w274 -> [w280 w295 w308 w353 w359]
            tunnel: [w280 w294 w308 w353 w359] -> w273
            tunnel: [TRUE _ _ _ _] -> w272
            tunnel: w271 -> [_ _ w316 _ _]
            tunnel: [_ _ _ w334 w354] -> _
            frame Default {
              # "Done"
            }
            frame 0 {
              w281 = FALSE ("AudUtil Running")
              w286 = FALSE ("Lnch")
              # "Init Controls"
              n121 = invoke on="SN" class="Str" method="Reinit To Default"() -> ()  [unwired: 3 in, 3 out]
              n122 = property on="Status" class="Str"("Text.BGColor"=u32 13816530) -> ()  [unwired: 2 in, 2 out]
              n123 = Unbundle By Name(w285) -> ("Log"=w298:refnum<class "Event Notification.lvclass">)
              n124 = local write "Status"("Initializing" ("Status")) -> ()
              n125 = local write "Main Tab"(0) -> ()
              n126 = local write "Control Tab"(0) -> ()
              n127 = local write "Result Data Tab"(0) -> ()
              n128 = call <vilib>:"Event Notification.Status Message.vi"("Log"=TRUE, "Level"=Event_Log.Log_Level."Verbose", "Message"="Reset - Initializing", "Event Notification in"=w298) -> ()  [unwired: 8 in]
              n129 = local read "TE"() -> (w282:bool)
              n130 = case shown="True" w282 {
                frame False {
                }
                frame True {
                  n131 = control-ref of="This VI"() -> (w302:refnum<vi>)
                  n132 = invoke class="VI" method="FP.Center"(reference=w302) -> (reference out=w301:refnum<vi>, error out=w300:errorcluster)  [unwired: 2 in, 1 out]
                  n133 = invoke class="VI" method="FP.Open"(reference=w301, error in=w300, "Activate"=TRUE ("Activate?"), "State"=T13."Minimized") -> ()  [unwired: 1 in, 5 out]
                }
              }
              n134 = Unbundle By Name(w295) -> ("FunctData"=w292:refnum<class "FunctDataMgr.lvclass">)
              n135 = Unbundle By Name(w285) -> ("Cfg.Dirs.Config"=w284:path)
              n136 = call "FunctDataMgr.Reset Data.vi"("FunctDataMgr in"=w292) -> ("FunctDataMgr out"=w293:refnum<class "FunctDataMgr.lvclass">)  [unwired: 9 in, 1 out]
              n137 = Build Path(base path=w284, name or relative path="Audio Sequences") -> ()  [unwired: 1 out]
              n138 = Bundle By Name(cluster=w295, "FunctData"=w293, "Lnch"=w286, "Remote Test"=w286) -> (w294:T28)
              n139 = property on="AudUtil Running" class="Bool (strict)"("Blinking"=w281) -> ()  [unwired: 2 in, 2 out]
              "AudUtil Running" <- w281
            }
            frame 1 {
              # "Test End and Test Reset tasks will initialize the controls of this app."
              # "Enqueue Tasks"
              # "Lock Controls until after initialization is completed"
              n140 = Flush Queue(queue=w316) -> (queue out=w319:refnum<queue>)  [unwired: 1 in, 2 out]
              n141 = call <vilib>:"Scheduler.Clear-Reset.vi"("Q In"=w319) -> ("Q Out"=w318:refnum<queue>)  [unwired: 9 in, 1 out]
              n142 = call "Error.Clear.vi"("Q In"=w318) -> ("Q Out"=w317:refnum<queue>)  [unwired: 9 in, 1 out]
              n143 = To Variant(anything=FALSE) -> (Variant=w321:variant)
              n144 = Unbundle By Name(w307) -> ("Cfg.Dirs.Config"=w306:path)
              n145 = Unbundle By Name(w307) -> ("Child Modules"=w309:cluster{"Name":string, "vi ref":refnum<vi>}[])
              n146 = call <vilib>:"Q.Enqueue App.vi"("Data1"=w321, "Task Name"="Lock Test Controls", "Q In"=w317) -> ("Q Out"=w311:refnum<queue>)  [unwired: 7 in, 1 out]
              n147 = Unbundle By Name(w308) -> ("Lnch"=w310:bool)
              n148 = property on="Abort" class="Bool"("DisabledEnum"=T15."Disabled and Grayed Out" ("Disabled")) -> ()  [unwired: 2 in, 2 out]
              n149 = case shown="False" w310 {
                tunnel: w309 -> [w327 _]
                frame False {
                  # "Reset Child Modules"
                  n150 = call "Module.Reset Children.vi"("Child Modules"=w327) -> ()  [unwired: 11 in]
                }
                frame True {
                  # "Do not reset at launch.\nThey are already reset"
                }
              }
              n151 = case shown="True" TRUE {
                tunnel: w306 -> [_ w324]
                frame False {
                }
                frame True {
                  n152 = call "AudioTest.Config, Deploy Config Files.vi"("SkipIfExists(F)/Overwrite(T)"=FALSE, "Config Folder"=w324) -> ("error out"=w325:errorcluster)  [unwired: 9 in]
                  n153 = call <vilib>:"Clear Errors.vi"("error in (no error)"=w325) -> ()  [unwired: 5 in, 2 out]
                }
              }
              n154 = for {
                shift-right: [w330] -> w312
                shift-left: _ -> [w331]
                tunnel: string[] ["Test End", "Test Reset"] -> [w328] mode=indexing
                shift-right: [w329] -> w313
                shift-left: w311 -> [w332]
                n155 = call <vilib>:"Q.Enqueue Task.vi"("Error In"=w331, "Task Name"=w328, "Q In"=w332) -> ("error out"=w330:errorcluster, "Q Out"=w329:refnum<queue>)  [unwired: 7 in]
              }
              n156 = call <vilib>:"Q.Enqueue App.vi"("Error In"=w312, "Task Name"="Initialization Done", "Q In"=w313) -> ()  [unwired: 7 in, 2 out]
            }
            frame 2 {
              w345 = "SoundCheck"
              n157 = local read "SoundCheck Config"() -> (w339:T3)
              n158 = Unbundle By Name(w352) -> ("Cfg.Dirs.Config"=w351:path)
              n159 = Build Path(base path=w351, name or relative path="Local Station.ini") -> (appended path=w349:path)
              n160 = Unbundle By Name(w339) -> ("SoundCheckApp"=w340:path, "Process Name"=w335:string)
              n161 = call <vilib>:"Open Config Data.vi"("configuration file path"=w349) -> ("error out"=w333:errorcluster, "refnum"=w348:T30)  [unwired: 8 in, 1 out]
              n162 = call-poly <vilib>:"Read Key.vi"("section"=w345, "error in (no error)"=w333, "default value"=w340, "key"="ExePath", "refnum"=w348) -> ("error out"=w343:errorcluster, "value"=w337:path, "refnum out"=w346:T30)  [unwired: 3 in, 1 out]
              n163 = call-poly <vilib>:"Read Key.vi"("section"=w345, "error in (no error)"=w343, "default value"=w335, "key"="ProcessName", "refnum"=w346) -> ("error out"=w341:errorcluster, "value"=w336:string, "refnum out"=w342:T30)  [unwired: 3 in, 1 out]
              n164 = call <vilib>:"Close Config Data.vi"("error in (no error)"=w341, "refnum"=w342) -> ("error out"=w334:errorcluster)  [unwired: 8 in, 1 out]
              n165 = Bundle By Name(cluster=w339, "SoundCheckApp"=w337, "Process Name"=w336) -> (w338:T3)
              n166 = local write "SoundCheck Config"(w338) -> ()
            }
            frame 3 {
              n167 = List Folder(path=path "C:/MTE/Audio Test/Config/SoundCheck/Sequences", pattern="*.sqc") -> (filenames=w355:string[], error out=w354:errorcluster)  [unwired: 2 in, 2 out]
              n168 = property on="Audio Seq Name" class="Ring (strict)"("Strings []"=w355) -> ()  [unwired: 2 in, 2 out]
            }
          }
        }
      }
      frame "Task" {
        n169 = case shown="\"Config - Reset Audio Limit Config\"" w365 {
          selector: w365 -> [_ _ _ _ _ _ _ _ _ _ _ _ _ _ _ _ _ _ w712 _ _ _ _ _ _ _ w805]
          tunnel: w369 -> [w384 w399 w404 w415 w429 w463 w477 w480 w492 w514 w530 w556 w592 w594 w607 w688 w696 w704 w713 w723 w729 w738 w740 w786 w788 w790 w813]
          tunnel: w368 -> [w375 w400 w410 w421 w428 w467 w473 w478 w491 w515 w524 w553 w589 w593 w606 w682 w691 w699 w707 w726 w728 w731 w747 w785 w787 w800 w808]
          tunnel: [w384 w399 w404 w415 w429 w463 w477 w480 w497 w514 w530 w556 w592 w594 w603 w688 w696 w704 w713 w722 w729 w738 w740 w786 w788 w790 w812] -> w367
          tunnel: [w374 w398 w410 w421 w428 w467 w472 w478 w491 w515 w523 w555 w588 w595 w602 w684 w693 w701 w706 w726 w728 w736 w741 w784 w787 w800 w807] -> w366
          tunnel: w364 -> [w387 w394 _ _ _ _ w476 _ w502 _ w528 _ w591 _ w604 w686 w695 w703 w710 w725 _ w737 w748 w783 _ w791 w810]
          tunnel: w363 -> [w388 _ _ _ _ _ _ _ w500 w517 _ w569 _ w598 w605 _ _ _ w711 _ _ _ _ _ _ _ _]
          tunnel: w362 -> [_ _ _ _ _ _ _ _ _ _ _ _ _ _ _ _ _ _ _ _ _ _ _ _ _ _ w815]
          tunnel: w361 -> [_ w393 _ _ _ _ _ _ _ _ _ _ _ _ _ _ _ _ _ _ _ _ _ _ _ _ w816]
          tunnel: [_ w395 _ _ w424 _ w475 w481 _ _ _ w552 _ _ w601 _ _ _ _ _ _ _ w743 _ _ _ w814] -> w360
          frame "Funct Local Call" {
            n170 = Variant To Data(type=string[] [], Variant=w387) -> (data=w378:string[])  [unwired: 1 in, 1 out]
            n171 = Delete From Array(array=w378, index=0) -> (deleted portion=w372:string, array with subset deleted=w376:string[])  [unwired: 1 in]
            n172 = Unbundle By Name(w384) -> ("Log"=w383:refnum<class "Event Notification.lvclass">)
            n173 = Concatenate Strings("Running: ", w372) -> (w382:string)
            n174 = call <vilib>:"Q.Enqueue Task.vi"("Task Name"="Test Start", "Q In"=w388) -> ("Q Out"=w391:refnum<queue>)  [unwired: 8 in, 1 out]
            n175 = call <vilib>:"Event Notification.Status Message.vi"("Level"=Event_Log.Log_Level."Verbose", "Message"=w382, "Event Notification in"=w383) -> ()  [unwired: 9 in]
            n176 = To Variant(anything=w376) -> (Variant=w371:variant)
            n177 = Get Date/Time In Seconds() -> (seconds since 1Jan1904=→"Start Time":timestamp)
            n178 = local write "Duration(s)"(0.0 ("Duration(s)")) -> ()
            n179 = call <vilib>:"Q.Enqueue Item.vi"("Data1"=w371, "Sub"=w372, "Cmd"="Function", "Q In"=w391) -> ("Q Out"=w390:refnum<queue>)  [unwired: 6 in, 1 out]
            n180 = call <vilib>:"Q.Enqueue Task.vi"("Task Name"="Test End", "Q In"=w390) -> ()  [unwired: 8 in, 2 out]
            n181 = Bundle By Name(cluster=w375, "Remote Test"=FALSE ("Local Test")) -> (w374:T28)
          }
          frame "Funct RTN" {
            n182 = Unbundle By Name(w400) -> ("FunctData"=w397:refnum<class "FunctDataMgr.lvclass">)
            n183 = call "FunctDataMgr.Function Return.vi"("RTN Info"=w393, "RTN Vars"=w394, "FunctDataMgr in"=w397) -> ("Error Out"=w395:errorcluster, "FunctDataMgr out"=w396:refnum<class "FunctDataMgr.lvclass">)  [unwired: 7 in]
            n184 = Bundle By Name(cluster=w400, "FunctData"=w396) -> (w398:T28)
          }
          frame "Module Undock - HMD" {
            n185 = Unbundle By Name(w404) -> ("Child Modules"=w402:cluster{"Name":string, "vi ref":refnum<vi>}[])
            n186 = control-ref of="HMDPanel"() -> (w405:refnum<vi>)
            n187 = Index Array(array=w402) -> (element=w403:cluster{"Name":string, "vi ref":refnum<vi>})  [unwired: 1 in]
            n188 = Unbundle By Name(w403) -> ("Name"=w401:string)
            n189 = call <vilib>:"Module.Window, Q Task.vi"("Sub Panel"=w405, "Q Name"=w401, "Action"=Window.Task,_Action."Dock to SubPanel(SubPanel Ref)") -> ("error out"=w407:errorcluster)  [unwired: 7 in, 1 out]
            n190 = call <vilib>:"Clear Errors.vi"("error in (no error)"=w407) -> ("error out"=w406:errorcluster)  [unwired: 5 in, 1 out]
            n191 = call <vilib>:"Module.Window, Q Task.vi"("Q Name"=w401, "error in"=w406, "Action"=Window.Task,_Action."Undock from SubPanel()") -> ()  [unwired: 7 in, 2 out]
          }
          frame "Module Undock - Servo" {
            n192 = Unbundle By Name(w415) -> ("Child Modules"=w413:cluster{"Name":string, "vi ref":refnum<vi>}[])
            n193 = control-ref of="ServoPanel"() -> (w416:refnum<vi>)
            n194 = Index Array(array=w413, index=2) -> (element=w414:cluster{"Name":string, "vi ref":refnum<vi>})
            n195 = Unbundle By Name(w414) -> ("Name"=w412:string)
            n196 = call <vilib>:"Module.Window, Q Task.vi"("Sub Panel"=w416, "Q Name"=w412, "Action"=Window.Task,_Action."Dock to SubPanel(SubPanel Ref)") -> ("error out"=w418:errorcluster)  [unwired: 7 in, 1 out]
            n197 = call <vilib>:"Clear Errors.vi"("error in (no error)"=w418) -> ("error out"=w417:errorcluster)  [unwired: 5 in, 1 out]
            n198 = call <vilib>:"Module.Window, Q Task.vi"("Q Name"=w412, "error in"=w417, "Action"=Window.Task,_Action."Undock from SubPanel()") -> ()  [unwired: 7 in, 2 out]
          }
          frame "Launch SoundCheck" {
            n199 = local read "SoundCheck Config"() -> (w423:T3)
            n200 = Unbundle By Name(w423) -> ("SoundCheckApp"=w426:path, "Process Name"=w425:string, "Window"=w422:enum16{"Normal", "Minimized", "Hidden"})
            n201 = call "System.Processes.vi"("Process Name"=w425) -> ("Is Running"=w427:bool)  [unwired: 8 in, 2 out]
            n202 = case shown="False" w427 {
              tunnel: [w435 _] -> w424
              tunnel: w426 -> [w434 _]
              tunnel: w423 -> [w433 _]
              tunnel: w422 -> [w430 _]
              frame False {
                n203 = call <vilib>:"File.Check if File or Folder Exists.vi"("Path"=w434) -> ("Exists"=w432:bool, "Dup Path"=w431:path)  [unwired: 6 in, 3 out]
                n204 = case shown="True" w432 {
                  tunnel: [w439 w451] -> w435
                  tunnel: w431 -> [_ w441]
                  tunnel: w433 -> [_ w450]
                  tunnel: w430 -> [_ w440]
                  frame False {
                    w436 = T29 -5400 items=["No Error"=0, "Abort"=-2, "Misc"=-5000, "Fixture Error"=-5100, "File IO - General"=-5200, "FIle IO - Config Error"=-5201, "Instrument - General"=-5300, "Instrument - Serial Com"=-5301, "Instrument - Camera"=-5302, "Instrument - PS"=-5303, "Instrument - Oscilloscope"=-5304, "Instrument - Function Gen"=-5305, "Instrument - Load"=-5306, "Instrument - Meter"=-5307, "Instrument - Power Control"=-5308, "Instrument - Motion"=-5309, "Instrument - RF"=-5310, "System Exe"=-5400, "Image Processing"=-5500, "Communication"=-5600, "Script - Syntax Error"=-6000, "Script - Invalid Name or Param"=-6100, "Script - Timeout"=-6200, "Invalid Data"=-6300, "FW Update Error"=-6500] ("Std Code")
                    n205 = call "Error.Set-Change Error Info.vi"("Std Code"=w436, "Description"="SoundCheck App does not exist.", "Set Error"=TRUE) -> ("error out"=w439:errorcluster)  [unwired: 8 in]
                  }
                  frame True {
                    w443 = "\"" ("string")
                    n206 = case shown="\"Hidden\"" w440 {
                      tunnel: ["" " -m" " -h"] -> w442
                      frame "Normal", Default {
                      }
                      frame "Minimized" {
                      }
                      frame "Hidden" {
                      }
                    }
                    n207 = Path To String(path=w441) -> (string=w444:string)
                    n208 = Concatenate Strings("cmd.exe /c ", w443, w444, w443, w442) -> (w449:string)
                    n209 = call <vilib>:"System Exec.vi"("run minimized? (F)"=TRUE, "wait until completion? (T)"=FALSE, "command line"=w449) -> ("error out"=w445:errorcluster)  [unwired: 5 in, 3 out]
                    n210 = case shown="No Error" w445 {
                      selector: w445 -> [_ w462]
                      tunnel: [w456 w462] -> w451
                      tunnel: w450 -> [w461 _]
                      frame No Error {
                        # "Wait for App to launch"
                        n211 = Unbundle By Name(w461) -> ("IP"=w460:string, "Port"=w459:u16)
                        n212 = call "SC TCP SoundCheck Wait for Ready.vi"("TimeOut(s)"=20.0, "port (4444)"=w459, "SoundCheck IP Address (localhost)"=w460) -> ("error out"=w457:errorcluster)  [unwired: 6 in, 2 out]
                        n213 = call <vilib>:"Time.Inline Delay.vi"("Wait(secs)"=0.1, "error in top"=w457) -> ("error out top"=w456:errorcluster)  [unwired: 8 in, 1 out]
                      }
                      frame Error {
                      }
                    }
                  }
                }
              }
              frame True {
                # "Do nothing\nAlready running"
              }
            }
          }
          frame "Config - Reset Audio Limit Config" {
            n214 = Unbundle By Name(w463) -> ("Cfg.Dirs.Config"=w465:path)
            n215 = call "AudioTest.Config, Deploy Config Files.vi"("SkipIfExists(F)/Overwrite(T)"=TRUE, "Config Folder"=w465) -> ("error out"=w466:errorcluster)  [unwired: 9 in]
            n216 = call <vilib>:"Clear Errors.vi"("error in (no error)"=w466) -> ()  [unwired: 5 in, 2 out]
          }
          frame "Set TimeOut" {
            n217 = Variant To Data(type=0.0, Variant=w476) -> (data=w470:dbl, error out=w475:errorcluster)  [unwired: 1 in]
            n218 = In Range and Coerce(upper limit=900.0, x=w470, lower limit=1.0) -> (coerced(x)=w471:dbl)  [unwired: 1 out]
            n219 = local write "Timeout(s)"(w471) -> ()
            n220 = Bundle By Name(cluster=w473, "Timeout(s)"=w471) -> (w472:T28)
          }
          frame "Report SW Ver" {
            n221 = Unbundle By Name(w480) -> ("SW Rev.AppName"=w484:string, "SW Rev.Version"=w483:string)
            n222 = Bundle By Name(cluster=T6 {"Name"="", "PN"="", "Version"="", "Note"=""} ("SW"), "Name"=w484, "Version"=w483) -> (w485:T6)
            n223 = Unbundle By Name(w480) -> ("Cfg.Is Child?"=w487:bool, "Cfg.Parent Q"=w482:refnum<queue>)
            n224 = Build Array(w485) -> (w479:T6[])
            n225 = case shown="False" w487 {
              tunnel: w482 -> [_ w490]
              tunnel: w479 -> [_ w489]
              tunnel: [_ w488] -> w481
              frame False {
              }
              frame True {
                n226 = call "TestExec.Client, SW Items.vi"("SW Items"=w489, "Q In"=w490) -> ("error out"=w488:errorcluster)  [unwired: 8 in, 1 out]
              }
            }
            n227 = local write "SW Items"(w479) -> ()
          }
          frame "TCP-IP" {
            n228 = Variant To Data(type=FALSE, Variant=w502) -> (data=w493:bool)  [unwired: 1 in, 1 out]
            n229 = Bundle By Name(cluster=w492, "Cfg.Is Child?"=w493) -> (w497:T12)
            n230 = case shown="True" w493 {
              tunnel: w500 -> [_ w508]
              tunnel: w491 -> [_ w504]
              frame False {
              }
              frame True {
                # "When Parent connects, Send SW Version and SW Framework Version"
                n231 = Unbundle By Name(w504) -> ("StaVer"=w503:i32)
                n232 = call <vilib>:"Q.Enqueue Task.vi"("Task Name"="Report SW Ver", "Q In"=w508) -> ("Q Out"=w507:refnum<queue>)  [unwired: 8 in, 1 out]
                n233 = To Variant(anything=w503) -> (Variant=w505:variant)
                n234 = call <vilib>:"Q.Enqueue Task.vi"("Data1"=w505, "Task Name"="Sta Notify Ver", "Q In"=w507) -> ()  [unwired: 7 in, 2 out]
              }
            }
            n235 = Unbundle By Name(w497) -> ("Log"=w499:refnum<class "Event Notification.lvclass">)
            n236 = Select(t="TCP-IP Connected", s=w493, f="TCP-IP Disconnected") -> (s? t:f=w494:string)
            n237 = call <vilib>:"Event Notification.Status Message.vi"("Level"=Event_Log.Log_Level."Verbose", "Message"=w494, "Event Notification in"=w499) -> ()  [unwired: 9 in]
          }
          frame "Abort", "Test Abort" {
            n238 = call <vilib>:"Scheduler.Clear-Reset.vi"("Q In"=w517) -> ("error out"=w519:errorcluster, "Q Out"=w518:refnum<queue>)  [unwired: 9 in]
            n239 = Flush Queue(queue=w518, error in (no error)=w519) -> (queue out=w516:refnum<queue>)  [unwired: 2 out]
            n240 = Unbundle By Name(w514) -> ("Log"=w513:refnum<class "Event Notification.lvclass">)
            n241 = for {
              N: 5 -> [_]
              n242 = call "Abort.Send Abort or Done Notificaiton.vi"("Abort(T)/Done(F)"=TRUE) -> ()  [unwired: 10 in, 1 out]
              n243 = Wait (ms)(milliseconds to wait=u32 10) -> ()  [unwired: 1 out]
            }
            n244 = call <vilib>:"Q.Enqueue Task.vi"("Task Name"="Test End", "Q In"=w516) -> ()  [unwired: 8 in, 2 out]
            n245 = call <vilib>:"Event Notification.Status Message.vi"("Level"=Event_Log.Log_Level."Verbose", "Message"="Test Aborted by Operator", "Event Notification in"=w513) -> ()  [unwired: 9 in]
          }
          frame "Test Data Dirs" {
            n246 = Variant To Data(type=T17[] [{"Name"="", "Path"=path ""}], Variant=w528) -> (data=w527:T17[])  [unwired: 1 in, 1 out]
            n247 = Unbundle By Name(w524) -> ("Dirs"=w526:T27)
            n248 = for {
              tunnel: w527 -> [w533] mode=indexing
              shift-right: [w534] -> w525
              shift-left: w526 -> [w535]
              n249 = Unbundle By Name(w533) -> ("Name"=w532:string, "Path"=w531:path)
              n250 = case shown="\"DataArchiveDir\"" w532 {
                tunnel: w535 -> [w536 w541 w546]
                tunnel: [w536 w540 w545] -> w534
                tunnel: w531 -> [_ w539 w544]
                tunnel: [_ _ w542] -> _
                tunnel: [_ w537 _] -> _
                frame Default {
                }
                frame "DataArchiveDir" {
                  n251 = call <vilib>:"File.Create Folder if Does Not Exist.vi"("Path"=w539) -> ("error out"=w537:errorcluster, "Dup Path"=w538:path)  [unwired: 8 in, 1 out]
                  n252 = Bundle By Name(cluster=w541, "Archive"=w538) -> (w540:T27)
                  n253 = local write "Archive Dir"(w538) -> ()
                }
                frame "DataSumArchiveDir" {
                  n254 = call <vilib>:"File.Create Folder if Does Not Exist.vi"("Path"=w544) -> ("error out"=w542:errorcluster, "Dup Path"=w543:path)  [unwired: 8 in, 1 out]
                  n255 = Bundle By Name(cluster=w546, "ArchiveSum"=w543) -> (w545:T27)
                  n256 = local write "Archive Summary Dir"(w543) -> ()
                }
              }
            }
            n257 = Bundle By Name(cluster=w524, "Dirs"=w525) -> (w523:T28)
          }
          frame "Test End" {
            w568 = FALSE
            n258 = Unbundle By Name(w556) -> ("Log"=w561:refnum<class "Event Notification.lvclass">)
            n259 = To Variant(anything=FALSE) -> (Variant=w572:variant)
            n260 = call <vilib>:"Q.Enqueue App.vi"("Top of Q"=TRUE, "Data1"=w572, "Task Name"="Lock Test Controls", "Q In"=w569) -> ()  [unwired: 6 in, 2 out]
            n261 = call <vilib>:"Event Notification.Status Message.vi"("Display"=TRUE, "Level"=Event_Log.Log_Level."Normal", "Message"="Test Completed.", "Event Notification in"=w561) -> ()  [unwired: 8 in]
            n262 = local read "UUT Dir"() -> (w548:path)
            n263 = property on="Test Reset" class="Bool"("DisabledEnum"=T15."Enabled" ("Disabled")) -> ()  [unwired: 2 in, 2 out]
            n264 = property on="Abort" class="Bool"("DisabledEnum"=T15."Disabled and Grayed Out" ("Disabled")) -> ()  [unwired: 2 in, 2 out]
            n265 = To Variant(anything=w548) -> (Variant=w549:variant)
            n266 = call <vilib>:"Q.Enqueue Task.vi"("Data1"=w549, "Q Name"="AudioGraphs", "Task Name"="Load Data") -> ()  [unwired: 7 in, 2 out]
            n267 = case shown="False" FALSE {
              tunnel: w553 -> [_ w574]
              tunnel: [_ w573] -> w552
              frame False {
              }
              frame True {
                # "Only do if is remote test.\nScript will handle this action"
                n268 = Unbundle By Name(w574) -> ("Dirs.UUTDir"=w575:path, "Dirs.Archive"=w577:path, "ResultState.State"=w578:T26)
                n269 = case shown="\"ERROR\"" w578 {
                  tunnel: [_ " - FAIL" " - ERROR" " - ABORT"] -> w576
                  frame "None", Default {
                  }
                  frame "Failing", "FAIL" {
                    (unwired) TRUE
                  }
                  frame "ERROR" {
                  }
                  frame "ABORT" {
                    (unwired) TRUE
                  }
                }
                n270 = call "File.Move to Archive Folder.vi"("NameSuffix"=w576, "ArchiveDir"=w577, "UUTDir"=w575) -> ("error out"=w573:errorcluster)  [unwired: 7 in, 1 out]
              }
            }
            n271 = property on="Test Running" class="Bool (strict)"("Blinking"=w568, "Value"=w568) -> ()  [unwired: 2 in, 2 out]
            n272 = Unbundle By Name(w556) -> ("Child Modules"=w557:cluster{"Name":string, "vi ref":refnum<vi>}[])
            n273 = local read "Start Time"() -> (w566:timestamp)
            n274 = Get Date/Time In Seconds() -> (seconds since 1Jan1904=w567:timestamp)
            n275 = for {
              tunnel: w557 -> [w582] mode=indexing
              n276 = Unbundle By Name(w582) -> ("Name"=w583:string)
              n277 = call <vilib>:"Q.Enqueue Task.vi"("Q Name"=w583, "Task Name"="Test End") -> ()  [unwired: 8 in, 2 out]
            }
            n278 = Bundle By Name(cluster=w553, "Remote Test"=FALSE) -> (w555:T28)
            n279 = Subtract(x=w567, y=w566) -> (x-y=→"Duration(s)":dbl)
          }
          frame "Test Mode" {
            # "TE will send the test mode at the start of a test.\nUse this to make decisions and/or to store with data.\nIt may not apply to this station module."
            n280 = Variant To Data(type="", Variant=w591) -> (data=w585:string)  [unwired: 1 in, 1 out]
            n281 = Unbundle By Name(w589) -> ("FunctData"=w587:refnum<class "FunctDataMgr.lvclass">)
            n282 = local write "Mode"(w585) -> ()
            n283 = call "FunctDataMgr.Update Test Mode.vi"("Mode"=w585, "FunctDataMgr in"=w587) -> ("FunctDataMgr out"=w586:refnum<class "FunctDataMgr.lvclass">)  [unwired: 8 in, 1 out]
            n284 = Bundle By Name(cluster=w589, "FunctData"=w586) -> (w588:T28)
          }
          frame "Test Reset" {
            n285 = call "Error.Clear.vi"("Q In"=w598) -> ()  [unwired: 9 in, 2 out]
            n286 = invoke on="Enumerated" class="Bool (strict)" method="Reinit To Default"() -> ()  [unwired: 3 in, 3 out]
            n287 = invoke on="Ran to completion" class="Bool (strict)" method="Reinit To Default"() -> ()  [unwired: 3 in, 3 out]
            n288 = invoke on="Duration(s)" class="DigNum (strict)" method="Reinit To Default"() -> ()  [unwired: 3 in, 3 out]
            n289 = property on="Status" class="Str"("Text.BGColor"=u32 13816530) -> ()  [unwired: 2 in, 2 out]
            n290 = local write "Status"("Idle") -> ()
            n291 = Unbundle By Name(w593) -> ("FunctData"=w596:refnum<class "FunctDataMgr.lvclass">)
            n292 = call "FunctDataMgr.Reset Data.vi"("FunctDataMgr in"=w596) -> ("FunctDataMgr out"=w597:refnum<class "FunctDataMgr.lvclass">)  [unwired: 9 in, 1 out]
            n293 = Bundle By Name(cluster=w593, "FunctData"=w597) -> (w595:T28)
          }
          frame "Test Start" {
            n294 = while {
              tunnel: w605 -> [w611]
              tunnel: w604 -> [w610]
              shift-right: [w614] -> w603
              shift-left: w607 -> [w616]
              shift-right: [w613] -> w602
              shift-left: w606 -> [w615]
              tunnel: [w608] -> w601
              i -> [w612]
              stop <- w609 stop-if-true
              n295 = case shown="3" w612 {
                tunnel: w616 -> [w630 w643 w659 w677 w680]
                tunnel: w615 -> [w620 w642 w655 w675 w679]
                tunnel: [w630 w643 w659 w677 w680] -> w614
                tunnel: [w622 w642 w655 w676 w679] -> w613
                tunnel: w611 -> [_ w640 w660 _ _]
                tunnel: w610 -> [w623 _ _ _ _]
                tunnel: [_ _ _ _ TRUE] -> w609
                tunnel: [errorcluster {"status"=FALSE, "code"=0, "source"=""} ("error constant") _ _ _ _] -> w608
                frame 0 {
                  # "Record Start Info"
                  n296 = Variant To Data(type=T18 {"Test Name"="", "Start Time"=timestamp(0 s since 1904-01-01), "UUT SN"=""} ("Test Start Info"), Variant=w623) -> (data=w629:T18, error out=w627:errorcluster)  [unwired: 1 in]
                  n297 = case shown="Error" w627 {
                    tunnel: w629 -> [w635 _]
                    tunnel: [w634 "Local" ("Test Name")] -> w628
                    tunnel: [w633 w636] -> w618
                    tunnel: [w632 w637] -> w619
                    tunnel: [TRUE _] -> w621
                    frame No Error {
                      # "Test launched from TE"
                      n298 = Unbundle By Name(w635) -> ("Test Name"=w634:string, "UUT SN"=w632:string, "Start Time"=w633:timestamp)
                      n299 = local write "Start Time"(w633) -> ()
                      n300 = local write "SN"(w632) -> ()
                    }
                    frame Error {
                      # "Test initiated locally"
                      n301 = local read "Start Time"() -> (w636:timestamp)
                      n302 = local read "SN"() -> (w637:string)
                    }
                  }
                  n303 = Unbundle By Name(w620) -> ("FunctData"=w626:refnum<class "FunctDataMgr.lvclass">)
                  n304 = call "FunctDataMgr.Test Start.vi"("Reset Data"=w621, "StartTime"=w618, "SN"=w619, "Sequence"=w628, "FunctDataMgr in"=w626) -> ("FunctDataMgr out"=w625:refnum<class "FunctDataMgr.lvclass">)  [unwired: 5 in, 1 out]
                  n305 = Bundle By Name(cluster=w620, "FunctData"=w625, "Remote Test"=w621) -> (w622:T28)
                }
                frame 1 {
                  w650 = TRUE
                  # "Init Controls"
                  n306 = call <vilib>:"Q.Enqueue Task.vi"("Top of Q"=TRUE, "Task Name"="Report SW Ver", "Q In"=w640) -> ()  [unwired: 7 in, 2 out]
                  n307 = property on="Test Reset" class="Bool"("DisabledEnum"=T15."Disabled and Grayed Out" ("Disabled")) -> ()  [unwired: 2 in, 2 out]
                  n308 = property on="Abort" class="Bool"("DisabledEnum"=T15."Enabled" ("Disabled")) -> ()  [unwired: 2 in, 2 out]
                  n309 = Unbundle By Name(w643) -> ("Log"=w649:refnum<class "Event Notification.lvclass">)
                  n310 = property on="Test Running" class="Bool (strict)"("Blinking"=w650) -> ()  [unwired: 2 in, 2 out]
                  n311 = call <vilib>:"Event Notification.Status Message with Error In.vi"("Display"=TRUE, "Log"=TRUE, "Level"=Event_Log.Log_Level."Verbose", "Type"=Event_Log.Notification_Type."Normal", "Message"="Test Running", "Event Notification in"=w649) -> ()  [unwired: 6 in]
                  "Test Running" <- w650
                }
                frame 2 {
                  # "Enqueue Tasks"
                  n312 = To Variant(anything=TRUE) -> (Variant=w664:variant)
                  n313 = Unbundle By Name(w655) -> ("Remote Test"=w654:bool)
                  n314 = local read "UUT Dir"() -> (w657:path)
                  n315 = call <vilib>:"Q.Enqueue App.vi"("Top of Q"=TRUE, "Data1"=w664, "Task Name"="Lock Test Controls", "Q In"=w660) -> ("Q Out"=w658:refnum<queue>)  [unwired: 6 in, 1 out]
                  n316 = Not A Number/Path/Refnum?(number/path/refnum=w657) -> (NaN/Path/Refnum?=w656:bool)
                  n317 = Or(x=w654, y=w656) -> ()  [unwired: 1 out]
                  n318 = case shown="False" FALSE {
                    tunnel: w658 -> [_ w667]
                    frame False {
                    }
                    frame True {
                      n319 = call <vilib>:"Q.Enqueue Task.vi"("Top of Q"=TRUE, "Task Name"="Init UUT Folder", "Q In"=w667) -> ()  [unwired: 7 in, 2 out]
                    }
                  }
                  n320 = Unbundle By Name(w659) -> ("Child Modules"=w665:cluster{"Name":string, "vi ref":refnum<vi>}[])
                  n321 = for {
                    tunnel: w665 -> [w670] mode=indexing
                    n322 = Unbundle By Name(w670) -> ("Name"=w671:string)
                    n323 = call <vilib>:"Q.Enqueue Task.vi"("Top of Q"=TRUE, "Q Name"=w671, "Task Name"="Test Start") -> ()  [unwired: 7 in, 2 out]
                  }
                }
                frame 3 {
                  # "Init Test Data"
                  n324 = Bundle By Name(cluster=w675, "Script"="", "Mic"=T20 {"State"=0, "Norm"=[0.0, 0.0, 0.0], "Covered"=[0.0, 0.0, 0.0]}) -> (w676:T28)
                }
                frame Default {
                  # "Done"
                }
              }
            }
          }
          frame "Test Attr Data" {
            n325 = Variant To Data(type=T21[] [] ("Data.Attr"), Variant=w686) -> (data=w685:T21[])  [unwired: 1 in, 1 out]
            n326 = Unbundle By Name(w682) -> ("FunctData"=w681:refnum<class "FunctDataMgr.lvclass">)
            n327 = call "FunctDataMgr.Update Attribute Data.vi"("Data.Attr"=w685, "FunctDataMgr in"=w681) -> ("FunctDataMgr out"=w683:refnum<class "FunctDataMgr.lvclass">)  [unwired: 8 in, 1 out]
            n328 = Bundle By Name(cluster=w682, "FunctData"=w683) -> (w684:T28)
          }
          frame "Test Num Data" {
            n329 = Variant To Data(type=T22[] [] ("data"), Variant=w695) -> (data=w694:T22[])  [unwired: 1 in, 1 out]
            n330 = Unbundle By Name(w691) -> ("FunctData"=w690:refnum<class "FunctDataMgr.lvclass">)
            n331 = call "FunctDataMgr.Update Numeric Data.vi"("Data.Num"=w694, "FunctDataMgr in"=w690) -> ("FunctDataMgr out"=w692:refnum<class "FunctDataMgr.lvclass">)  [unwired: 8 in, 1 out]
            n332 = Bundle By Name(cluster=w691, "FunctData"=w692) -> (w693:T28)
          }
          frame "Test Meas Data" {
            n333 = Variant To Data(type=T4[] [] ("data"), Variant=w703) -> (data=w702:T4[])  [unwired: 1 in, 1 out]
            n334 = Unbundle By Name(w699) -> ("FunctData"=w698:refnum<class "FunctDataMgr.lvclass">)
            n335 = call "FunctDataMgr.Update Meas Data.vi"("Data.Meas"=w702, "FunctDataMgr in"=w698) -> ("FunctDataMgr out"=w700:refnum<class "FunctDataMgr.lvclass">)  [unwired: 8 in, 1 out]
            n336 = Bundle By Name(cluster=w699, "FunctData"=w700) -> (w701:T28)
          }
          frame "Result - Measurements" {
            n337 = call <vilib>:"Q.Enqueue Task.vi"("Task Name"="Update Results", "Q In"=w711) -> ()  [unwired: 8 in, 2 out]
            n338 = Variant To Data(type=T4[] [] ("Data.MeasData"), Variant=w710) -> (data=w705:T4[])  [unwired: 1 in, 1 out]
            n339 = Unbundle By Name(w713) -> ("Cfg.Parent Q"=w715:refnum<queue>)
            n340 = Not A Number/Path/Refnum?(number/path/refnum=w715) -> (NaN/Path/Refnum?=w714:bool)
            n341 = case shown="False" w714 {
              tunnel: w712 -> [w720 _]
              tunnel: w710 -> [w719 _]
              tunnel: w715 -> [w718 _]
              frame False {
                n342 = call <vilib>:"Q.Enqueue Task.vi"("Data1"=w719, "Task Name"=w720, "Q In"=w718) -> ()  [unwired: 7 in, 2 out]
              }
              frame True {
              }
            }
            n343 = Unbundle By Name(w707) -> ("FunctData"=w709:refnum<class "FunctDataMgr.lvclass">)
            n344 = call "FunctDataMgr.Function Add RTN Data.vi"("Meas"=w705, "FunctDataMgr in"=w709) -> ("FunctDataMgr out"=w708:refnum<class "FunctDataMgr.lvclass">)  [unwired: 9 in]
            n345 = Bundle By Name(cluster=w707, "FunctData"=w708) -> (w706:T28)
          }
          frame "Set Config" {
            n346 = Unbundle By Name(w723) -> ("AppData"=w724:refnum<class "Class.AppData.lvclass">)
            n347 = call <vilib>:"ClassAppData.Load_Merge Data.vi"("Data In"=w725, "Class - App Data in"=w724) -> ("Class - App Data out"=w721:refnum<class "Class.AppData.lvclass">)  [unwired: 8 in, 1 out]
            n348 = Bundle By Name(cluster=w723, "AppData"=w721) -> (w722:T12)
          }
          frame "Update Results" {
            n349 = Unbundle By Name(w728) -> ("FunctData"=w727:refnum<class "FunctDataMgr.lvclass">)
            n350 = call "FunctDataMgr.Update Result Table Value.vi"("FunctDataMgr in"=w727) -> ()  [unwired: 9 in, 2 out]
          }
          frame "Test Status" {
            w735 = T25 {"State"=enum."Passing", "Code"=0, "Description"=""}  # ResultState
            n351 = Variant To Data(type=w735, Variant=w737) -> (data=w730:T25)  [unwired: 1 in, 1 out]
            n352 = Unbundle By Name(w731) -> ("FunctData"=w733:refnum<class "FunctDataMgr.lvclass">)
            n353 = call "FunctDataMgr.Update Result State.vi"("Result Info"=w730, "FunctDataMgr in"=w733) -> ("FunctDataMgr out"=w734:refnum<class "FunctDataMgr.lvclass">)  [unwired: 8 in, 1 out]
            n354 = Bundle By Name(cluster=w731, "FunctData"=w734) -> (w732:T28)
            n355 = Bundle By Name(cluster=w732, "ResultState"=w730) -> (w736:T28)
          }
          frame "Update SN" {
            n356 = Variant To Data(type="", Variant=w748) -> (data=w744:string)  [unwired: 1 in, 1 out]
            n357 = Unbundle By Name(w747) -> ("FunctData"=w751:refnum<class "FunctDataMgr.lvclass">)
            n358 = Unbundle By Name(w747) -> ("Dirs.UUTDir"=w746:path)
            n359 = local write "SN"(w744) -> ()
            n360 = call "FunctDataMgr.Update SN.vi"("SN"=w744, "FunctDataMgr in"=w751) -> ("FunctDataMgr out"=w750:refnum<class "FunctDataMgr.lvclass">)  [unwired: 8 in, 1 out]
            n361 = call <vilib>:"File.Check if File or Folder Exists.vi"("Path"=w746) -> ("Dup Path"=w745:path)  [unwired: 6 in, 4 out]
            n362 = Bundle By Name(cluster=w747, "FunctData"=w750) -> (w742:T28)
            n363 = case shown="True" FALSE {
              tunnel: w745 -> [_ w758]
              tunnel: w744 -> [_ w767]
              tunnel: [_ w765] -> w743
              tunnel: w742 -> [w752 w764]
              tunnel: [w752 w763] -> w741
              tunnel: w740 -> [_ w754]
              frame False {
              }
              frame True {
                # "Replace SN"
                n364 = Strip Path(path=w758) -> (stripped path=w757:path, name=w769:string)
                n365 = Match Pattern(string=w769, regular expression="_") -> (match substring=w759:string, after substring=w760:string)  [unwired: 1 in, 2 out]
                n366 = Concatenate Strings(w767, w759, w760) -> (w766:string)
                n367 = Build Path(base path=w757, name or relative path=w766) -> (appended path=w762:path)
                n368 = Not Equal?(x=w758, y=w762) -> (x != y?=w761:bool)
                n369 = Unbundle By Name(w754) -> ("Cfg.Parent Q"=w756:refnum<queue>)
                n370 = case shown="True" w761 {
                  tunnel: [_ w780] -> w765
                  tunnel: [w776 w779] -> w753
                  tunnel: w758 -> [w776 w778]
                  tunnel: w762 -> [_ w777]
                  frame False {
                  }
                  frame True {
                    n371 = Move(source path=w778, 10:w777) -> (error out=w780:errorcluster, 3:w779:path)  [unwired: 3 in, 1 out]
                  }
                }
                n372 = Not A Number/Path/Refnum?(number/path/refnum=w756) -> (NaN/Path/Refnum?=w755:bool)
                n373 = local write "UUT Dir"(w753) -> ()
                n374 = case shown="False" w755 {
                  tunnel: w756 -> [w775 _]
                  tunnel: w753 -> [w771 _]
                  frame False {
                    n375 = Path To String(path=w771) -> (string=w774:string)
                    n376 = Build Array("UUTDir", w774) -> (w773:string[])
                    n377 = Build Array(w773) -> (w770:string[][])
                    n378 = call "TestExec.Set Seq Variable.vi"("Variables"=w770, "Q In"=w775) -> ()  [unwired: 9 in, 1 out]
                  }
                  frame True {
                  }
                }
                n379 = Bundle By Name(cluster=w764, "Dirs.UUTDir"=w753) -> (w763:T28)
              }
            }
          }
          frame "Update UUT Folder" {
            n380 = Variant To Data(type=path "", Variant=w783) -> (data=w781:path)  [unwired: 1 in, 1 out]
            n381 = Bundle By Name(cluster=w785, "Dirs.UUTDir"=w781) -> (w784:T28)
            n382 = local write "UUT Dir"(w781) -> ()
          }
          frame "Sta Notify Ver" {
          }
          frame "Warning" {
            n383 = Variant To Data(type=errorcluster {"status"=FALSE, "code"=0, "source"=""} ("error constant"), Variant=w791) -> (data=w792:errorcluster)  [unwired: 1 in, 1 out]
            n384 = Unbundle By Name(w790) -> ("Cfg.Is Child?"=w799:bool, "Cfg.Parent Q"=w798:refnum<queue>)
            n385 = case shown="True" w799 {
              tunnel: w798 -> [_ w802]
              tunnel: w792 -> [_ w803]
              tunnel: [_ w804] -> _
              frame False {
              }
              frame True {
                n386 = call "TestExec.Health Status, Set Error_Warning.vi"("error in"=w803, "Health State Cmd"=TestExec.Health_State_Command."Set Warning", "Q In"=w802) -> ("error out"=w804:errorcluster)  [unwired: 8 in]
              }
            }
            n387 = Unbundle By Name(w792) -> ("source"=w795:string)
            n388 = Concatenate Strings("WARNING: ", w795) -> (w796:string)
            n389 = Bundle By Name(cluster=w792, "status"=FALSE, "source"=w796) -> (w789:errorcluster)
            n390 = local write "Error"(w789) -> ()
          }
          frame Default {
            # "Handle default function tasks"
            n391 = Unbundle By Name(w808) -> ("FunctData"=w811:refnum<class "FunctDataMgr.lvclass">)
            n392 = call "FunctDataMgr.Default Tasks.vi"("Data In"=w810, "Task In"=w805, "FunctDataMgr in"=w811) -> ("Not Fwd Data"=w806:bool, "FunctDataMgr out"=w809:refnum<class "FunctDataMgr.lvclass">)  [unwired: 6 in, 1 out]
            n393 = case shown="True" w806 {
              tunnel: w816 -> [_ w829]
              tunnel: w815 -> [w818 w828]
              tunnel: [w818 w827] -> w814
              tunnel: w813 -> [w819 w826]
              tunnel: [w819 w825] -> w812
              tunnel: w810 -> [_ w824]
              tunnel: w809 -> [w817 _]
              tunnel: w808 -> [w821 w823]
              tunnel: [w820 w823] -> w807
              tunnel: w805 -> [_ w822]
              frame False {
                # "Task Handled"
                n394 = Bundle By Name(cluster=w821, "FunctData"=w817) -> (w820:T28)
              }
              frame True {
                # "Handle default module tasks"
                n395 = call <vilib>:"Module.Default Tasks.vi"("Sys"=w826, "error in"=w828, "Data2"=w829, "Data1"=w824, "Sub"=w822) -> ("error out"=w827:errorcluster, "Sys Out"=w825:T12)  [unwired: 5 in]
              }
            }
          }
        }
      }
      frame "Function" {
        n396 = while {
          shift-right: [w851] -> w837
          shift-left: w839 -> [w852]
          shift-right: [w849] -> w836
          shift-left: w838 -> [w850]
          shift-right: [w847] -> _
          shift-left: _ -> [w848]
          shift-right: [w844] -> w834
          shift-left: w835 -> [w845]
          tunnel: w833 -> [w843]
          tunnel: w832 -> [w842]
          tunnel: w831 -> [w841]
          tunnel: w830 -> [w840]
          i -> [w853]
          stop <- w846 stop-if-true
          n397 = case shown="1" w853 {
            tunnel: w852 -> [w858 w877 w1180]
            tunnel: [w858 w875 w1180] -> w851
            tunnel: w850 -> [w866 w876 w1178]
            tunnel: [w865 w874 w1177] -> w849
            tunnel: w848 -> [_ _ w1174]
            tunnel: [FALSE w869 _] -> w847
            tunnel: [_ _ TRUE] -> w846
            tunnel: w845 -> [_ w868 w1175]
            tunnel: [_ w872 w1176] -> w844
            tunnel: w843 -> [w857 w873 _]
            tunnel: w842 -> [_ w871 w1173]
            tunnel: w841 -> [_ w870 _]
            tunnel: w840 -> [w863 _ _]
            frame 0 {
              # "Default to Immediate Return"
              # "Init"
              n398 = Unbundle By Name(w866) -> ("FunctData"=w867:refnum<class "FunctDataMgr.lvclass">)
              n399 = call "FunctDataMgr.Function Initialize.vi"("RTN Info"=w863, "Name"=w857, "FunctDataMgr in"=w867) -> ("FunctDataMgr out"=w864:refnum<class "FunctDataMgr.lvclass">)  [unwired: 7 in, 1 out]
              n400 = Bundle By Name(cluster=w866, "FunctData"=w864) -> (w865:T28)
              n401 = Format Into String(format string="Performing: %s", w857) -> (resulting string=w859:string)  [unwired: 2 in, 1 out]
              n402 = Unbundle By Name(w858) -> ("Log"=w861:refnum<class "Event Notification.lvclass">)
              n403 = call <vilib>:"Event Notification.Status Message.vi"("Display"=TRUE ("Log"), "Log"=FALSE, "Level"=Event_Log.Log_Level."Verbose", "Message"=w859, "Event Notification in"=w861) -> ()  [unwired: 7 in]
            }
            frame 1 {
              # "Execute"
              n404 = case shown="\"RunAudioCheckUtil\"" w873 {
                selector: w873 -> [_ _ _ _ _ _ _ _ _ _ _ _ _ _ w1166]
                tunnel: w877 -> [w891 w900 w930 w952 w974 w994 w1005 w1010 w1016 w1074 w1088 w1116 w1130 w1142 w1164]
                tunnel: w876 -> [w882 w913 w938 w963 w968 w995 w1004 w1009 w1019 w1063 w1093 w1115 w1124 w1140 w1162]
                tunnel: [w891 w900 w930 w952 w974 w994 w1005 w1010 w1016 w1074 w1088 w1116 w1130 w1142 w1164] -> w875
                tunnel: [w879 w912 w937 w962 w976 w996 w1004 w1009 w1047 w1075 w1093 w1115 w1125 w1140 w1172] -> w874
                tunnel: [_ _ _ _ _ _ _ _ _ w1068 _ w1105 _ w1138 w1159] -> w872
                tunnel: w871 -> [_ w895 _ w948 _ _ w1003 _ _ _ _ _ _ _ w1168]
                tunnel: w870 -> [_ w894 w924 w947 w980 _ _ _ _ _ _ w1109 w1126 w1139 w1165]
                tunnel: [_ _ _ _ _ _ _ _ _ _ _ _ _ _ FALSE] -> w869
                tunnel: w868 -> [_ _ _ _ _ _ _ _ _ _ _ _ _ _ w1167]
                frame "Create_UUTFolder" {
                  n405 = Unbundle By Name(w882) -> ("Dirs.Temp Data"=w885:path)
                  n406 = local read "SN"() -> (w884:string)
                  n407 = local read "Start Time"() -> (w883:timestamp)
                  n408 = call "File.Create UUT Dir.vi"("Start Time"=w883, "SN"=w884, "Local Data Dir"=w885) -> ("error out"=w878:errorcluster, "UUTDir"=w880:path)  [unwired: 6 in, 1 out]
                  n409 = local write "UUT Dir"(w880) -> ()
                  n410 = Path To String(path=w880) -> (string=w888:string)
                  n411 = Build Array("UUTDir", w888) -> (w886:string[])
                  n412 = Unbundle By Name(w882) -> ("FunctData"=w890:refnum<class "FunctDataMgr.lvclass">)
                  n413 = Build Array(w886) -> (w881:string[][])
                  n414 = call "FunctDataMgr.Function Add RTN Data.vi"("Vars"=w881, "Error In"=w878, "FunctDataMgr in"=w890) -> ("FunctDataMgr out"=w889:refnum<class "FunctDataMgr.lvclass">)  [unwired: 8 in]
                  n415 = Bundle By Name(cluster=w882, "FunctData"=w889, "Dirs.UUTDir"=w880) -> (w879:T28)
                }
                frame "GetUUTSN_OLD" {
                  n416 = Unbundle By Name(w900) -> ("Child Modules"=w899:cluster{"Name":string, "vi ref":refnum<vi>}[])
                  n417 = local read "Timeout(s)"() -> (w904:dbl)
                  n418 = Index Array(array=w899) -> (element=w898:cluster{"Name":string, "vi ref":refnum<vi>})  [unwired: 1 in]
                  n419 = Unbundle By Name(w898) -> ("Name"=w897:string)
                  n420 = Multiply(x=w904, y=1000.0 ("x")) -> (x*y=w907:dbl)
                  n421 = To Long Integer(number=w907) -> (32bit integer=w906:i32)
                  n422 = call <vilib>:"Q.Send Function Command and wait on Ret Data.vi"("Timeout(ms)"=w906, "Q Name"=w897, "Data1"=w894, "Cmd"="CfgReadTopSN", "Q In"=w895) -> ("error out"=w892:errorcluster, "Ret"=w910:variant)  [unwired: 5 in]
                  n423 = Variant To Data(type=string[][] [], Variant=w910) -> (data=w908:string[][], error out=w909:errorcluster)  [unwired: 1 in]
                  n424 = case shown="No Error" w909 {
                    tunnel: w908 -> [w922 _]
                    tunnel: [w922 _] -> w893
                    frame No Error {
                    }
                    frame Error {
                    }
                  }
                  n425 = case shown="No Error" w892 {
                    tunnel: w893 -> [w921 _]
                    tunnel: [w918 _] -> w901
                    frame No Error {
                      n426 = Index Array(array=w921, index (row)=0, index (col)=1 ("disabled index (col)")) -> (element=w918:string)
                    }
                    frame Error {
                    }
                  }
                  n427 = Unbundle By Name(w913) -> ("FunctData"=w915:refnum<class "FunctDataMgr.lvclass">)
                  n428 = Empty String/Path?(string/path=w901) -> (empty?=w902:bool)
                  n429 = case shown="True" w902 {
                    tunnel: w901 -> [w916 _]
                    tunnel: [w916 ""] -> w896
                    frame False {
                    }
                    frame True {
                    }
                  }
                  n430 = call "FunctDataMgr.Function Add RTN Data.vi"("Vars"=w893, "Error In"=w892, "FunctDataMgr in"=w915) -> ("FunctDataMgr out"=w914:refnum<class "FunctDataMgr.lvclass">)  [unwired: 8 in]
                  n431 = Bundle By Name(cluster=w913, "FunctData"=w914) -> (w912:T28)
                  n432 = local write "SN"(w896) -> ()
                }
                frame "GetUUTSN" {
                  n433 = Variant To Data(type=string[] [], Variant=w924) -> (data=w925:string[], error out=w926:errorcluster)  [unwired: 1 in]
                  n434 = Unbundle By Name(w930) -> ("Child Modules"=w936:cluster{"Name":string, "vi ref":refnum<vi>}[])
                  n435 = case shown="No Error" w926 {
                    tunnel: w925 -> [w942 _]
                    tunnel: [w941 _] -> w923
                    frame No Error {
                      n436 = Index Array(array=w942) -> (element=w941:string)  [unwired: 1 in]
                    }
                    frame Error {
                    }
                  }
                  n437 = Index Array(array=w936) -> (element=w935:cluster{"Name":string, "vi ref":refnum<vi>})  [unwired: 1 in]
                  n438 = Unbundle By Name(w930) -> ("Cfg.Parent Q"=w934:refnum<queue>, "Cfg.Is Child?"=w933:bool)
                  n439 = Unbundle By Name(w935) -> ("Name"=w929:string)
                  n440 = call "TestExec.HMD, Pull SN from UUT.vi"("VarName"=w923, "ParentQ"=w934, "HMD Q Name"=w929, "IsChild"=w933) -> ("error out"=w928:errorcluster, "Vars"=w931:string[][], "SN"=w932:string)  [unwired: 5 in]
                  n441 = case shown="No Error" w928 {
                    tunnel: w932 -> [w943 _]
                    frame No Error {
                      n442 = local write "SN"(w943) -> ()
                    }
                    frame Error {
                    }
                  }
                  n443 = Unbundle By Name(w938) -> ("FunctData"=w940:refnum<class "FunctDataMgr.lvclass">)
                  n444 = call "FunctDataMgr.Function Add RTN Data.vi"("Vars"=w931, "Error In"=w928, "FunctDataMgr in"=w940) -> ("FunctDataMgr out"=w939:refnum<class "FunctDataMgr.lvclass">)  [unwired: 8 in]
                  n445 = Bundle By Name(cluster=w938, "FunctData"=w939) -> (w937:T28)
                }
                frame "CheckUutEnumStatus" {
                  n446 = Unbundle By Name(w952) -> ("Child Modules"=w951:cluster{"Name":string, "vi ref":refnum<vi>}[])
                  n447 = local read "Timeout(s)"() -> (w954:dbl)
                  n448 = Index Array(array=w951) -> (element=w950:cluster{"Name":string, "vi ref":refnum<vi>})  [unwired: 1 in]
                  n449 = Unbundle By Name(w950) -> ("Name"=w949:string)
                  n450 = Multiply(x=w954, y=1000.0 ("x")) -> (x*y=w957:dbl)
                  n451 = To Long Integer(number=w957) -> (32bit integer=w956:i32)
                  n452 = call <vilib>:"Q.Send Function Command and wait on Ret Data.vi"("Timeout(ms)"=w956, "Q Name"=w949, "Data1"=w947, "Cmd"="GetEnumStatus", "Q In"=w948) -> ("error out"=w946:errorcluster, "Ret"=w960:variant)  [unwired: 5 in]
                  n453 = Variant To Data(type=string[][] [], Variant=w960) -> (data=w958:string[][], error out=w959:errorcluster)  [unwired: 1 in]
                  n454 = case shown="No Error" w959 {
                    tunnel: w958 -> [w966 _]
                    tunnel: [w966 _] -> w945
                    frame No Error {
                    }
                    frame Error {
                    }
                  }
                  n455 = call "Hmd.Check RtnVars for Enumerated Status.vi"("Vars"=w945) -> ("Enumerated"=→"Enumerated":bool)  [unwired: 2 in]
                  n456 = Unbundle By Name(w963) -> ("FunctData"=w965:refnum<class "FunctDataMgr.lvclass">)
                  n457 = call "FunctDataMgr.Function Add RTN Data.vi"("Vars"=w945, "Error In"=w946, "FunctDataMgr in"=w965) -> ("FunctDataMgr out"=w964:refnum<class "FunctDataMgr.lvclass">)  [unwired: 8 in]
                  n458 = Bundle By Name(cluster=w963, "FunctData"=w964) -> (w962:T28)
                }
                frame "RunAudioScript" {
                  n459 = Variant To Data(type=string[] [], Variant=w980) -> (data=w981:string[], error out=w982:errorcluster)  [unwired: 1 in]
                  n460 = case shown="No Error" w982 {
                    tunnel: w981 -> [w984 _]
                    tunnel: [w984 _] -> w979
                    frame No Error {
                    }
                    frame Error {
                    }
                  }
                  n461 = Index Array(array=w979) -> (element=w967:string)  [unwired: 1 in]
                  n462 = local read "Timeout(s)"() -> (w972:dbl)
                  n463 = Bundle By Name(cluster=w968, "Script"=w967) -> (w969:T28)
                  n464 = local read "UUT Dir"() -> (w971:path)
                  n465 = property on="Audio Seq Name" class="Ring (strict)"("RingText.Text"=w967) -> ()  [unwired: 2 in, 2 out]
                  n466 = call "AudioTest.Run SoundCheck Sequence.vi"("Config"="SoundCheck Config", "UUT Dir"=w971, "Timeout(s)"=w972, "Sequence"=w967) -> ("error out"=w975:errorcluster, "Ran to completion"=→"Ran to completion":bool)  [unwired: 4 in, 2 out]
                  n467 = Unbundle By Name(w969) -> ("FunctData"=w978:refnum<class "FunctDataMgr.lvclass">)
                  n468 = call "FunctDataMgr.Function Add RTN Data.vi"("Error In"=w975, "FunctDataMgr in"=w978) -> ("FunctDataMgr out"=w977:refnum<class "FunctDataMgr.lvclass">)  [unwired: 9 in]
                  n469 = Bundle By Name(cluster=w969, "FunctData"=w977) -> (w976:T28)
                }
                frame "RunAudioCheckUtil" {
                  n470 = flat-sequence {
                    tunnel: [errorcluster {"status"=FALSE, "code"=0, "source"=""} ("error constant")] -> w990
                    frame #0 {
                      w1000 = TRUE ("AudUtil Running")
                      n471 = invoke on="Audio Util Check" class="Clust (strict)" method="Reinit To Default"() -> ()  [unwired: 3 in, 3 out]
                      n472 = invoke on="Audio Utuil Dur(s)" class="DigNum (strict)" method="Reinit To Default"() -> ()  [unwired: 3 in, 3 out]
                      n473 = property on="AudUtil Running" class="Bool (strict)"("Value"=w1000, "Blinking"=w1000) -> ()  [unwired: 2 in, 2 out]
                    }
                  }
                  n474 = Unbundle By Name(w994) -> ("Cfg.Dirs.Config"=w993:path)
                  n475 = call <vilib>:"Time.Inline Record Start Time Secs.vi"("Error In Upper"=w990) -> ("Start(s)"=w986:dbl, "Error Out Upper"=w989:errorcluster)  [unwired: 8 in, 1 out]
                  n476 = call "AudioTest, Audio Test Util, Manager.vi"("error in (no error)"=w989, "Config Folder"=w993) -> ("Error Out"=w988:errorcluster, "Meas"=w992:T4)  [unwired: 6 in, 2 out]
                  "Audio Util Check" <- w992
                  n477 = call <vilib>:"Time.Inline Calculate Duration Secs.vi"("Start(Sec)"=w986, "Error In Top"=w988) -> ("Duration(s)"=→"Audio Utuil Dur(s)":dbl, "Error Out Top"=w987:errorcluster)  [unwired: 7 in, 1 out]
                  n478 = Build Array(w992) -> (w991:T4[])
                  n479 = Unbundle By Name(w995) -> ("FunctData"=w998:refnum<class "FunctDataMgr.lvclass">)
                  n480 = flat-sequence {
                    tunnel: w987 -> [_]
                    frame #0 {
                      w1001 = FALSE ("AudUtil Running")
                      n481 = property on="AudUtil Running" class="Bool (strict)"("Value"=w1001, "Blinking"=w1001) -> ()  [unwired: 2 in, 2 out]
                    }
                  }
                  n482 = call "FunctDataMgr.Function Add RTN Data.vi"("Error In"=w988, "Meas"=w991, "FunctDataMgr in"=w998) -> ("FunctDataMgr out"=w997:refnum<class "FunctDataMgr.lvclass">)  [unwired: 8 in]
                  n483 = Bundle By Name(cluster=w995, "FunctData"=w997) -> (w996:T28)
                }
                frame "SoundCheckLaunch" {
                  n484 = call <vilib>:"Q.Enqueue Task.vi"("Task Name"="Launch SoundCheck", "Q In"=w1003) -> ()  [unwired: 8 in, 2 out]
                }
                frame "SoundCheckKill" {
                  n485 = local read "SoundCheck Config"() -> (w1007:T3)
                  n486 = Unbundle By Name(w1007) -> ("Process Name"=w1008:string)
                  n487 = call "System.Processes.vi"("Kill"=TRUE, "Process Name"=w1008) -> ()  [unwired: 7 in, 3 out]
                }
                frame "ParseAudioResults" {
                  # "Get Results\n  Produce Num Results\nGet Plots\n  Look up Plot Limits\n  Evaluate P/F\n  Produce Attribute Results"
                  n488 = Unbundle By Name(w1019) -> ("Script"=w1026:string)
                  n489 = Unbundle By Name(w1016) -> ("Cfg.Dirs.Config"=w1015:path)
                  n490 = local read "UUT Dir"() -> (w1045:path)
                  n491 = Concatenate Strings(w1026, "*_results.txt" ("Primary Search String")) -> (w1028:string)
                  n492 = Concatenate Strings(w1026, "*_data.txt" ("pattern")) -> (w1025:string)
                  n493 = List Folder(path=w1045, pattern=w1025) -> (path out=w1033:path, filenames=w1035:string[])  [unwired: 2 in, 2 out]
                  n494 = call "AudioTest.Config - Read Plot Analysis Params.vi"("Config Dir"=w1015) -> ("Avg(F)/Float(T)"=w1014:bool, "End Freq"=w1011:dbl, "Start Freq"=w1013:dbl)  [unwired: 8 in]
                  n495 = Unbundle By Name(w1019) -> ("Mic.Norm"=w1023:dbl[], "Mic.State"=w1021:u16)
                  n496 = Index Array(array=w1035) -> (element=w1034:string)  [unwired: 1 in]
                  n497 = Build Array(w1013, w1011) -> (w1012:dbl[])
                  n498 = Build Path(base path=w1033, name or relative path=w1034) -> (appended path=w1032:path)
                  n499 = To Long Integer(number=w1021) -> (32bit integer=w1022:i32)
                  n500 = call "AudioTest.SoundCheck Data Log Analysis_Module - Load Data Task.vi"("Q Name"="AudioGraphs", "UUT Folder"=w1045) -> ("error out"=w1042:errorcluster)  [unwired: 9 in]
                  n501 = Build Path(base path=w1015, name or relative path="SoundCheck Graph Definitions.csv") -> (appended path=→"Graph Def File":path)
                  n502 = call "AudioTest.Parse SoundCheck Results File.vi"("SoundCheck Mic Data Name"="LEFT_MIC_SENSITIVITY" ("SoundCheckData Name"), "Primary Search String"=w1028, "Config Dir"=w1015, "Results Folder"=w1045) -> ("error out"=w1031:errorcluster, "Name Lookup"=→"Name Lookup":variant, "Mic"=w1017:dbl, "Meas"=w1037:T4[], "Lookup File"=→"Name Lookup File":path)  [unwired: 3 in]
                  n503 = call "AudioTest.Parse SoundCheck Data Log TXT File.vi"("Lim Center at Average(f), Float at center"=w1014, "Start_End"=w1012, "Config Folder"=w1015, "SoundCheck Data File"=w1032) -> ("error out"=w1030:errorcluster, "Meas Rslt"=w1036:T4[])  [unwired: 4 in, 2 out]
                  n504 = Replace Array Subset(array=w1023, new element=w1017, index=w1022) -> (w1024:dbl[])
                  n505 = call <vilib>:"Clear Errors.vi"("error in (no error)"=w1042) -> ()  [unwired: 5 in, 2 out]
                  n506 = Bundle By Name(cluster=w1019, "Mic.Norm"=w1024) -> (w1020:T28)
                  n507 = Unbundle By Name(w1020) -> ("FunctData"=w1049:refnum<class "FunctDataMgr.lvclass">)
                  n508 = Build Array (concatenate)(w1036, w1037) -> (w1046:T4[])
                  n509 = Merge Errors(w1031, w1030) -> (w1044:errorcluster)
                  n510 = call "FunctDataMgr.Function Add RTN Data.vi"("Error In"=w1044, "Meas"=w1046, "FunctDataMgr in"=w1049) -> ("FunctDataMgr out"=w1048:refnum<class "FunctDataMgr.lvclass">)  [unwired: 8 in]
                  n511 = Bundle By Name(cluster=w1020, "FunctData"=w1048) -> (w1047:T28)
                }
                frame "ParseMicrophoneCoveredResults" {
                  n512 = Unbundle By Name(w1063) -> ("Script"=w1072:string)
                  n513 = local read "UUT Dir"() -> (w1073:path)
                  n514 = Unbundle By Name(w1063) -> ("Mic.Covered"=w1070:dbl[], "Mic.State"=w1069:u16, "Mic.Norm"=w1062:dbl[])
                  n515 = for {
                    N: 3 -> [_]
                    tunnel: w1073 -> [w1085]
                    tunnel: w1072 -> [w1084]
                    tunnel: [w1083] -> w1068
                    tunnel: [w1082] -> w1059
                    tunnel: [w1079] -> w1055
                    tunnel: "Covered Mic Level" ("Measurement Name") -> [w1081]
                    tunnel: string[] ["LEFT_MIC_SEAL_SENSITIVITY", "LEFT_MIC_SENSITIVITY", "Covered Mic Level"] -> [w1080] mode=indexing
                    stop <- w1078 stop-if-true
                    n516 = call "AudioTest.Parse Sealed Mic Result.vi"("Measurement Name"=w1081, "SoundCheckData Name(s)"=w1080, "Seq Name"=w1084, "Result Folder"=w1085) -> ("error out"=w1083:errorcluster, "Found"=w1078:bool, "Mic Level"=w1082:dbl, "Meas"=w1079:T4[])  [unwired: 4 in]
                  }
                  n517 = To Long Integer(number=w1069) -> (32bit integer=w1061:i32)
                  n518 = Index Array(array=w1062, index=w1061) -> (element=w1060:dbl)
                  n519 = Replace Array Subset(array=w1070, new element=w1059, index=w1061) -> (w1071:dbl[])
                  n520 = Subtract(x=w1060, y=w1059) -> (x-y=w1058:dbl)
                  n521 = Bundle By Name(cluster=w1063, "Mic.Covered"=w1071) -> (w1064:T28)
                  n522 = Number To Fractional String(number=w1058, precision (6)=i16 3) -> (F-format string=w1057:string)  [unwired: 2 in]
                  n523 = Bundle By Name(cluster=T4 {"Cnt"=0, "Step"="", "Category"="", "Name"="", "Value"="", "Units"="", "LimType"="", "LL"="", "UL"="", "Status"=0, "Code"=0, "Desc"="", "Time"=timestamp(0 s since 1904-01-01)} ("Meas"), "Category"="Mic", "Name"="Mic Gasket Attenuation" ("Category"), "Value"=w1057) -> (w1054:T4)
                  n524 = Unbundle By Name(w1064) -> ("FunctData"=w1077:refnum<class "FunctDataMgr.lvclass">)
                  n525 = Build Array (concatenate)(w1055, w1054) -> (w1053:T4[])
                  n526 = call "FunctDataMgr.Function Add RTN Data.vi"("Meas"=w1053, "FunctDataMgr in"=w1077) -> ("FunctDataMgr out"=w1076:refnum<class "FunctDataMgr.lvclass">)  [unwired: 9 in]
                  n527 = Bundle By Name(cluster=w1064, "FunctData"=w1076) -> (w1075:T28)
                }
                frame "AnalyzeData" {
                  # "SendDataToSta()\n  Sta.AnalyzeData()"
                  n528 = Unbundle By Name(w1088) -> ("Cfg.Dirs.Config"=w1087:path)
                  n529 = Unbundle By Name(w1088) -> ("Cfg.Parent Q"=w1091:refnum<queue>)
                  n530 = Unbundle By Name(w1093) -> ("FunctData"=w1092:refnum<class "FunctDataMgr.lvclass">)
                  n531 = call "FunctDataMgr.Read Result Data.vi"("FunctDataMgr in"=w1092) -> ("Result Info"=w1090:T25, "Meas"=w1086:T4[])  [unwired: 5 in, 4 out]
                  n532 = Unbundle By Name(w1090) -> ("State"=w1089:T26)
                  n533 = case shown="Default" w1089 {
                    tunnel: w1091 -> [_ w1098]
                    tunnel: w1086 -> [_ w1097]
                    tunnel: w1087 -> [_ w1094]
                    frame "ABORT", "ERROR" {
                      # "Do Nothing"
                    }
                    frame Default {
                      n534 = call "Results.Evaluate Overall Result Based on Failure Priority.vi"("ConfigDir"=w1094, "Meas"=w1097) -> ("Change"=w1095:bool, "Result Info"=w1096:T25)  [unwired: 8 in]
                      n535 = case shown="True" w1095 {
                        tunnel: w1098 -> [_ w1101]
                        tunnel: w1096 -> [_ w1099]
                        frame False {
                        }
                        frame True {
                          n536 = local read "TE"() -> (w1100:bool)
                          n537 = case shown="True" w1100 {
                            tunnel: w1099 -> [_ w1104]
                            tunnel: [_ w1103] -> _
                            tunnel: w1101 -> [_ w1102]
                            frame False {
                            }
                            frame True {
                              n538 = call "TestExec.Result, Overwrite Test Result State.vi"("ResultState"=w1104, "Q In"=w1102) -> ("error out"=w1103:errorcluster)  [unwired: 9 in]
                            }
                          }
                        }
                      }
                    }
                  }
                }
                frame "Archive_Results" {
                  n539 = Unbundle By Name(w1115) -> ("Dirs.UUTDir"=w1114:path, "Dirs.Archive"=w1113:path, "ResultState.State"=w1107:T26)
                  n540 = Variant To Data(type=string[] [], Variant=w1109) -> (data=w1110:string[], error out=w1111:errorcluster)  [unwired: 1 in]
                  n541 = case shown="No Error" w1111 {
                    tunnel: w1110 -> [w1120 _]
                    tunnel: [w1120 _] -> w1108
                    frame No Error {
                    }
                    frame Error {
                    }
                  }
                  n542 = case shown="\"Failing\", \"FAIL\"" w1107 {
                    tunnel: [_ " - FAIL" " - ERROR" " - ABORT"] -> w1106
                    frame "None", Default {
                    }
                    frame "Failing", "FAIL" {
                      (unwired) TRUE
                    }
                    frame "ERROR" {
                    }
                    frame "ABORT" {
                      (unwired) TRUE
                    }
                  }
                  n543 = call "File.Move to Archive Folder.vi"("NameSuffix"=w1106, "SubDirList"=w1108, "ArchiveDir"=w1113, "UUTDir"=w1114) -> ("error out"=w1105:errorcluster)  [unwired: 6 in, 1 out]
                }
                frame "SetMicState" {
                  n544 = Variant To Data(type=string[] [], Variant=w1126) -> (data=w1127:string[], error out=w1128:errorcluster)  [unwired: 1 in]
                  n545 = case shown="No Error" w1128 {
                    tunnel: w1127 -> [w1134 _]
                    tunnel: [w1134 _] -> w1123
                    frame No Error {
                    }
                    frame Error {
                    }
                  }
                  n546 = Index Array(array=w1123) -> (element=w1122:string)  [unwired: 1 in]
                  n547 = case shown="\"1\", \"Left\"" w1122 {
                    tunnel: [u16 1 ("AudioTestInfo.MicState") u16 2 ("AudioTestInfo.MicState") u16 0 ("AudioTestInfo.MicState")] -> w1121
                    frame "1", "Left" {
                    }
                    frame "2", "Right" {
                    }
                    frame "0", "Both", Default {
                    }
                  }
                  n548 = Bundle By Name(cluster=w1124, "Mic.State"=w1121) -> (w1125:T28)
                }
                frame "Archive_SummaryResults" {
                  n549 = Unbundle By Name(w1140) -> ("Dirs.UUTDir"=w1137:path, "Dirs.ArchiveSum"=w1141:path)
                  n550 = call <vilib>:"File.Check if File or Folder Exists.vi"("Path"=w1137) -> ("Exists"=w1135:bool, "Dup Path"=w1136:path)  [unwired: 6 in, 3 out]
                  n551 = case shown="True" w1135 {
                    tunnel: w1141 -> [_ w1145]
                    tunnel: w1139 -> [_ w1154]
                    tunnel: w1136 -> [_ w1153]
                    tunnel: [_ w1147] -> w1138
                    frame False {
                    }
                    frame True {
                      w1151 = T29 -5200 items=["No Error"=0, "Abort"=-2, "Misc"=-5000, "Fixture Error"=-5100, "File IO - General"=-5200, "FIle IO - Config Error"=-5201, "Instrument - General"=-5300, "Instrument - Serial Com"=-5301, "Instrument - Camera"=-5302, "Instrument - PS"=-5303, "Instrument - Oscilloscope"=-5304, "Instrument - Function Gen"=-5305, "Instrument - Load"=-5306, "Instrument - Meter"=-5307, "Instrument - Power Control"=-5308, "Instrument - Motion"=-5309, "Instrument - RF"=-5310, "System Exe"=-5400, "Image Processing"=-5500, "Communication"=-5600, "Script - Syntax Error"=-6000, "Script - Invalid Name or Param"=-6100, "Script - Timeout"=-6200, "Invalid Data"=-6300, "FW Update Error"=-6500] ("Std Code")
                      # "Need to separate adn group data to summary results if applicable."
                      n552 = Variant To Data(type=string[] [], Variant=w1154) -> (data=w1155:string[], error out=w1156:errorcluster)  [unwired: 1 in]
                      n553 = case shown="No Error" w1156 {
                        tunnel: w1155 -> [w1158 _]
                        tunnel: [w1158 _] -> w1144
                        frame No Error {
                        }
                        frame Error {
                        }
                      }
                      n554 = call "File.Build Path, Add Multiple Subfolders, Check for invalid Characters.vi"("Check/Create Dir"=TRUE, "Subfolders"=w1144, "Folder"=w1145) -> ("New Path"=w1143:path)  [unwired: 6 in, 2 out]
                      n555 = call <vilib>:"File.Create Folder if Does Not Exist.vi"("Path"=w1143) -> ("Dup Path"=w1149:path)  [unwired: 8 in, 2 out]
                      n556 = Move(source path=w1153, 10:w1149) -> (error out=w1152:errorcluster)  [unwired: 3 in, 2 out]
                      n557 = Format Into String(format string="Error archiving data.| Destination folder: \"%s\".", w1149) -> (resulting string=w1148:string)  [unwired: 2 in, 1 out]
                      n558 = call "Error.Set-Change Error Info.vi"("Std Code"=w1151, "error in"=w1152, "Description"=w1148) -> ("error out"=w1147:errorcluster)  [unwired: 8 in]
                    }
                  }
                }
                frame Default {
                  n559 = Unbundle By Name(w1164) -> ("Child Modules"=w1163:cluster{"Name":string, "vi ref":refnum<vi>}[])
                  n560 = Unbundle By Name(w1162) -> ("Timeout(s)"=w1161:dbl)
                  n561 = call "Function.Handle Default Case.vi"("Timeout(s)"=w1161, "Child Modules"=w1163, "Error In"=w1167, "Data1 In"=w1165, "Funct Name"=w1166, "Q In"=w1168) -> ("RTN Error"=w1159:errorcluster, "RTN Vars"=w1160:string[][])  [unwired: 4 in]
                  n562 = Unbundle By Name(w1162) -> ("FunctData"=w1170:refnum<class "FunctDataMgr.lvclass">)
                  n563 = call "FunctDataMgr.Function Add RTN Data.vi"("Vars"=w1160, "FunctDataMgr in"=w1170) -> ("FunctDataMgr out"=w1169:refnum<class "FunctDataMgr.lvclass">)  [unwired: 9 in]
                  n564 = Bundle By Name(cluster=w1162, "FunctData"=w1169) -> (w1172:T28)
                }
              }
            }
            frame Default {
              # "Return"
              n565 = case shown="False" w1174 {
                tunnel: w1178 -> [w1185 w1187]
                tunnel: [w1184 w1188] -> w1177
                tunnel: [w1182 _] -> w1176
                tunnel: w1175 -> [w1181 w1189]
                tunnel: w1173 -> [_ _]
                frame False {
                  n566 = Unbundle By Name(w1185) -> ("FunctData"=w1186:refnum<class "FunctDataMgr.lvclass">)
                  n567 = call "FunctDataMgr.Function Return.vi"("Error In"=w1181, "FunctDataMgr in"=w1186) -> ("Error Out"=w1182:errorcluster, "FunctDataMgr out"=w1183:refnum<class "FunctDataMgr.lvclass">)  [unwired: 8 in]
                  n568 = Bundle By Name(cluster=w1185, "FunctData"=w1183) -> (w1184:T28)
                }
                frame True {
                  # "In case, record error.\n\nThis case is reached when a function is set to retrn later (after some tasks have been performed.\nThat function(or one of its tasks) is responsible for enquing the 'Funct RTN' task."
                  n569 = Unbundle By Name(w1187) -> ("FunctData"=w1191:refnum<class "FunctDataMgr.lvclass">)
                  n570 = call "FunctDataMgr.Function Add RTN Data.vi"("Error In"=w1189, "FunctDataMgr in"=w1191) -> ("FunctDataMgr out"=w1190:refnum<class "FunctDataMgr.lvclass">)  [unwired: 9 in]
                  n571 = Bundle By Name(cluster=w1187, "FunctData"=w1190) -> (w1188:T28)
                }
              }
            }
          }
        }
      }
      frame "App" {
        n572 = case shown="\"Lock Test Controls\"" w1199 {
          tunnel: w1198 -> [_ _ w1220 _]
          tunnel: w1197 -> [_ w1202 _ w1232]
          tunnel: w1196 -> [_ _ _ _]
          tunnel: w1195 -> [w1201 w1207 w1225 w1235]
          tunnel: w1194 -> [w1200 w1206 w1224 w1233]
          tunnel: [w1201 w1207 w1225 w1228] -> w1193
          tunnel: [w1200 w1206 w1224 w1233] -> w1192
          frame Default {
          }
          frame "Lock Test Controls" {
            n573 = Variant To Data(type=FALSE, Variant=w1202) -> (data=w1204:bool, error out=w1205:errorcluster)  [unwired: 1 in]
            n574 = case shown="No Error" w1205 {
              selector: w1205 -> [_ w1219]
              tunnel: w1204 -> [w1212 _]
              tunnel: [_ w1219] -> _
              frame No Error {
                n575 = case shown="True" w1212 {
                  tunnel: [T15."Enabled" ("Disabled") T15."Disabled and Grayed Out" ("Disabled")] -> w1208
                  tunnel: [T15."Enabled" ("Disabled") T15."Disabled" ("Disabled")] -> _
                  tunnel: [TRUE ("Enable") FALSE ("Enable")] -> w1209
                  frame False {
                  }
                  frame True {
                  }
                }
                n576 = Current VI's Menubar() -> (w1210:refnum<k9>)
                n577 = call <vilib>:"Menu.Enable Item.vi"("Enable"=w1209, "Tag"="Config", "Menu Ref"=w1210) -> ()  [unwired: 7 in, 2 out]
                n578 = property on="Mode" class="Str"("DisabledEnum"=w1208) -> ()  [unwired: 2 in, 2 out]
                n579 = property on="SN" class="Str"("DisabledEnum"=w1208) -> ()  [unwired: 2 in, 2 out]
                n580 = property on="Get Top SN" class="Bool"("DisabledEnum"=w1208) -> ()  [unwired: 2 in, 2 out]
                n581 = property on="Archive Results" class="Bool"("DisabledEnum"=w1208) -> ()  [unwired: 2 in, 2 out]
                n582 = property on="Init UUT Folder" class="Bool"("DisabledEnum"=w1208) -> ()  [unwired: 2 in, 2 out]
                n583 = property on="Run SoundCheck Script" class="Bool"("DisabledEnum"=w1208) -> ()  [unwired: 2 in, 2 out]
                n584 = property on="Check UUT Enum Status" class="Bool"("DisabledEnum"=w1208) -> ()  [unwired: 2 in, 2 out]
                n585 = property on="Parse Results" class="Bool"("DisabledEnum"=w1208) -> ()  [unwired: 2 in, 2 out]
              }
              frame Error {
              }
            }
          }
          frame "Initialization Done" {
            n586 = To Variant(anything=FALSE) -> (Variant=w1222:variant)
            n587 = call <vilib>:"Q.Enqueue App.vi"("Data1"=w1222, "Task Name"="Lock Test Controls", "Q In"=w1220) -> ()  [unwired: 7 in, 2 out]
          }
          frame "Set Logging Level" {
            n588 = Variant To Data(type=Event_Log.Log_Level."Normal" ("Logging Level"), Variant=w1232) -> (data=w1226:T7)  [unwired: 1 in, 1 out]
            n589 = local read "Logging Level"() -> (w1229:T7)
            n590 = Unbundle By Name(w1235) -> ("Log"=w1234:refnum<class "Event Notification.lvclass">)
            n591 = call <vilib>:"Event Notification.Set Logging Level.vi"("Log Level"=w1226, "Event Notification in"=w1234) -> ("Event Notification out"=w1236:refnum<class "Event Notification.lvclass">)  [unwired: 9 in]
            n592 = Not Equal?(x=w1226, y=w1229) -> (x != y?=w1230:bool)
            n593 = case shown="True" w1230 {
              tunnel: w1226 -> [_ w1242]
              frame False {
              }
              frame True {
                n594 = local write "Logging Level"(w1242) -> ()
              }
            }
            n595 = Bundle By Name(cluster=w1235, "Log"=w1236) -> (w1228:T12)
            n596 = Unbundle By Name(w1228) -> ("Child Modules"=w1227:cluster{"Name":string, "vi ref":refnum<vi>}[])
            n597 = for {
              tunnel: w1227 -> [w1241] mode=indexing
              tunnel: w1226 -> [w1237]
              n598 = Unbundle By Name(w1241) -> ("Name"=w1238:string)
              n599 = To Variant(anything=w1237) -> (Variant=w1239:variant)
              n600 = call <vilib>:"Q.Enqueue App.vi"("Data1"=w1239, "Q Name"=w1238, "Task Name"="Set Logging Level") -> ()  [unwired: 7 in, 2 out]
            }
          }
        }
      }
      frame "Error", Default {
        n601 = case shown="\"Error\"" w1245 {
          selector: w1245 -> [_ w1288]
          tunnel: [_ w1289] -> w1248
          tunnel: w1243 -> [w1260 _]
          tunnel: w1244 -> [w1258 _]
          tunnel: w1246 -> [w1259 _]
          tunnel: w1247 -> [w1257 _]
          tunnel: w1251 -> [w1254 w1287]
          tunnel: w1250 -> [w1255 _]
          tunnel: [w1253 w1287] -> w1249
          frame "Error" {
            n602 = case shown="Default" w1259 {
              tunnel: w1260 -> [_ w1285 _]
              tunnel: w1258 -> [w1281 _ _]
              tunnel: [w1281 w1283 _] -> w1252
              tunnel: w1257 -> [w1280 w1282 w1286]
              tunnel: [w1280 w1282 w1286] -> w1256
              frame Default {
              }
              frame "Error" {
                n603 = Variant To Data(type=errorcluster {"status"=FALSE, "code"=0, "source"=""} ("error constant"), Variant=w1285) -> (data=w1283:errorcluster)  [unwired: 1 in, 1 out]
              }
              frame "Clear" {
              }
            }
            n604 = case shown="Error" w1252 {
              selector: w1252 -> [_ w1276]
              tunnel: w1256 -> [_ _]
              tunnel: w1255 -> [w1264 w1274]
              tunnel: w1254 -> [w1262 w1270]
              tunnel: [w1262 w1270] -> w1253
              frame No Error {
                # "Clear Local Errors"
                n605 = local read "Error"() -> (w1261:errorcluster)
                n606 = Unbundle By Name(w1264) -> ("Log"=w1263:refnum<class "Event Notification.lvclass">)
                n607 = case shown="Error" w1261 {
                  tunnel: w1263 -> [_ w1269]
                  frame No Error {
                  }
                  frame Error {
                    n608 = invoke on="Error" class="Clust (strict)" method="Reinit To Default"() -> ()  [unwired: 3 in, 3 out]
                    n609 = call <vilib>:"Event Notification.Status Message.vi"("Log"=TRUE, "Level"=Event_Log.Log_Level."Verbose", "Message"="Cleared Errors", "Event Notification in"=w1269) -> ()  [unwired: 8 in]
                  }
                }
                n610 = control-ref of="Error Status"() -> (w1265:refnum<vi>)
                n611 = call <vilib>:"Status.Simple Text Status Indicator.vi"("Status TextBox"=w1265) -> ()  [unwired: 10 in, 1 out]
              }
              frame Error {
                # "Record Error"
                n612 = Unbundle By Name(w1274) -> ("Log"=w1273:refnum<class "Event Notification.lvclass">)
                n613 = Unbundle By Name(w1276) -> ("code"=w1278:i32, "source"=w1277:string)
                n614 = Format Into String(format string="ERROR!!! Code: %d, Desc: %s", w1278, w1277) -> (resulting string=w1272:string)  [unwired: 2 in, 1 out]
                n615 = control-ref of="Error Status"() -> (w1275:refnum<vi>)
                n616 = call <vilib>:"Event Notification.Status Message with Error In.vi"("Type"=Event_Log.Notification_Type."Error", "Message"=w1272, "Event Notification in"=w1273) -> ()  [unwired: 9 in]
                n617 = call <vilib>:"Status.Simple Text Status Indicator.vi"("error in"=w1276, "Status TextBox"=w1275) -> ()  [unwired: 9 in, 1 out]
                "Error" <- w1276
              }
            }
          }
          frame Default {
            n618 = Concatenate Strings("Undefined State: \"", w1288, "\".") -> (w1290:string)
            n619 = Bundle By Name(cluster=errorcluster {"status"=TRUE, "code"=-5000, "source"=""} ("error constant"), "source"=w1290) -> (w1289:errorcluster)
          }
        }
      }
      frame "Exit" {
        # "This connection is made to not close\n the module until exit tasks are done."
        n620 = stacked-sequence {
          tunnel: w1298 -> [_ _ _]
          tunnel: [errorcluster {"status"=FALSE, "code"=0, "source"=""} ("error constant") _ _] -> w1297
          tunnel: [_ w1309 _] -> _
          tunnel: [_ w1307 _] -> _
          tunnel: w1294 -> [w1302 _ w1311]
          tunnel: [_ _ w1313] -> _
          frame #0 {
            # "Close connection to instruments"
            n621 = Unbundle By Name(w1302) -> ("Child Modules"=w1301:cluster{"Name":string, "vi ref":refnum<vi>}[])
            n622 = for {
              tunnel: w1301 -> [w1306] mode=indexing
              tunnel: [w1304] -> _ mode=indexing
              n623 = Unbundle By Name(w1306) -> ("Name"=w1305:string)
              n624 = call <vilib>:"Q.Enqueue Exit.vi"("Q Name"=w1305) -> ("error out"=w1304:errorcluster)  [unwired: 9 in, 1 out]
            }
          }
          frame #1 {
            n625 = call <vilib>:"Q.Enqueue Exit.vi"("Q Name"="Graphs" ("Control Q")) -> ("error out"=w1307:errorcluster)  [unwired: 9 in, 1 out]
            n626 = call <vilib>:"Q.Enqueue Exit.vi"("Q Name"="TCP-IP_Bridge" ("Control Q")) -> ("error out"=w1309:errorcluster)  [unwired: 9 in, 1 out]
          }
          frame #2 {
            w1317 = "SoundCheck"
            n627 = local read "SoundCheck Config"() -> (w1319:T3)
            n628 = Unbundle By Name(w1311) -> ("Cfg.Dirs.Config"=w1325:path)
            n629 = Unbundle By Name(w1319) -> ("SoundCheckApp"=w1320:path, "Process Name"=w1318:string)
            n630 = Build Path(base path=w1325, name or relative path="Local Station.ini") -> (appended path=w1324:path)
            n631 = call <vilib>:"Open Config Data.vi"("configuration file path"=w1324) -> ("error out"=w1327:errorcluster, "refnum"=w1323:T30)  [unwired: 8 in, 1 out]
            n632 = call-poly <vilib>:"Write Key.vi"("section"=w1317, "error in (no error)"=w1327, "value"=w1320, "key"="ExePath", "refnum"=w1323) -> ("error out"=w1321:errorcluster, "refnum out"=w1322:T30)  [unwired: 4 in, 1 out]
            n633 = call-poly <vilib>:"Write Key.vi"("section"=w1317, "error in (no error)"=w1321, "value"=w1318, "key"="ProcessName", "refnum"=w1322) -> ("error out"=w1326:errorcluster, "refnum out"=w1312:T30)  [unwired: 4 in, 1 out]
            n634 = call <vilib>:"Close Config Data.vi"("error in (no error)"=w1326, "refnum"=w1312) -> ("error out"=w1313:errorcluster)  [unwired: 8 in, 1 out]
          }
        }
        n635 = Bundle By Name(cluster=w1294, "Cfg.Is Child?"=FALSE) -> (w1295:T12)
        n636 = call <vilib>:"Module.Destructor.vi"("error in"=w1297, "Sys"=w1295) -> ("error out"=w1300:errorcluster)  [unwired: 9 in]
      }
    }
  }
  n637 = while "Event Loop" {
    tunnel: w1 -> [w1331]
    stop <- w1332 stop-if-true
    n638 = Unbundle By Name(w1331) -> ("Stop.Ref"=w1330:refnum<event-registration>, "Main Q"=w1329:refnum<queue>)
    n639 = event shown="[13] \"Run Audio Check\": Value Change" {
      selector: w1330 -> [_ _ _ _ _ _ _ _ _ _ _ _ _ _ _ _ _ _ _ _ _ _ _ _ _ _ _ _]
      dyn-events: _ -> [_ _ _ _ _ _ _ _ _ _ _ _ _ _ _ _ _ _ _ _ _ _ _ _ _ _ _ _]
      timeout: 1000 -> [_ _ _ _ _ _ _ _ _ _ _ _ _ _ _ _ _ _ _ _ _ _ _ _ _ _ _ _]
      tunnel: [w1335 TRUE w1351 _ _ _ _ _ _ _ _ _ _ _ _ _ _ _ _ _ _ _ _ _ _ _ _ _] -> w1332
      tunnel: w1331 -> [w1334 _ w1349 _ _ _ _ _ _ _ _ _ _ _ _ _ _ _ _ _ _ _ _ _ _ _ _ _]
      tunnel: w1329 -> [w1337 _ w1350 w1374 _ _ w1384 w1388 w1394 w1396 w1402 w1407 w1413 w1418 w1423 w1428 w1430 w1436 w1442 _ w1458 w1462 w1470 w1476 w1489 w1505 w1510 _]
      event Panel Close? {
        n640 = event-data() -> ()  [unwired: 1 in, 4 out]
        n641 = Unbundle By Name(w1334) -> ("Cfg.Is Child?"=w1333:bool)
        n642 = case shown="True" w1333 {
          tunnel: w1337 -> [w1340 w1343]
          tunnel: [TRUE TRUE] -> w1336
          tunnel: [TRUE FALSE] -> w1335
          tunnel: [_ w1341] -> _
          frame False {
            # "Parent - Exit"
            n643 = call <vilib>:"Q.Enqueue Exit.vi"("Q In"=w1340) -> ()  [unwired: 9 in, 2 out]
          }
          frame True {
            # "Child - Hide Panel and if was \nin a subpanel, return to subpanel."
            n644 = call <vilib>:"Module.Window, Q Task.vi"("Action"=Window.Task,_Action."Return to SubPanel()", "Q In"=w1343) -> ("error out"=w1341:errorcluster)  [unwired: 8 in, 1 out]
          }
        }
        n645 = event-data("Discard?"=w1336) -> ()  [unwired: 1 in, 1 out]
      }
      event User Event {
        n646 = event-data() -> ()  [unwired: 1 in, 5 out]
      }
      event Menu Selection (User) {
        n647 = event-data() -> ("MenuRef"=w1347:refnum<k9>, "ItemTag"=w1348:string)  [unwired: 1 in, 5 out]
        n648 = case shown="\"Help.About\"" w1348 {
          selector: w1348 -> [w1353 _ _ _ _ w1363 _ _]
          tunnel: [_ TRUE _ _ _ _ _ _] -> w1351
          tunnel: w1350 -> [_ w1356 _ w1359 _ w1367 w1369 w1372]
          tunnel: [_ _ w1358 _ _ _ _ _] -> _
          tunnel: w1349 -> [w1352 _ _ _ w1361 _ _ _]
          tunnel: w1347 -> [_ _ _ _ _ w1364 _ _]
          frame Default {
            # "Check if a help document was selected.\nIf so, open the document"
            n649 = Unbundle By Name(w1352) -> ("Docs.Tags"=w1355:string[], "Docs.Paths"=w1354:path[])
            n650 = call <vilib>:"Menu.Help, Open User Manual Items.vi"("Menu Tag Selection"=w1353, "Paths"=w1354, "Tags"=w1355) -> ()  [unwired: 8 in, 1 out]
          }
          frame "Exit" {
            n651 = call <vilib>:"Q.Enqueue Exit.vi"("Q In"=w1356) -> ()  [unwired: 9 in, 2 out]
          }
          frame "Event Log" {
            n652 = call <vilib>:"Event Log.Show.vi"() -> ("error out"=w1358:errorcluster)  [unwired: 11 in]
          }
          frame "Reset" {
            n653 = call <vilib>:"Q.Enqueue Reset.vi"("Q In"=w1359) -> ()  [unwired: 9 in, 2 out]
          }
          frame "Help.About" {
            n654 = Unbundle By Name(w1361) -> ("SW Rev"=w1360:T11)
            n655 = call <vilib>:"Help.About.vi"("SW Version"=w1360) -> ()  [unwired: 11 in]
          }
          frame "Simulate OFF", "Simulate ON" {
            n656 = call <vilib>:"Menu.Simulate, Set Menu State.vi"("Menu Tag"=w1363, "Menu Ref"=w1364) -> ("Sim ON"=w1362:bool)  [unwired: 8 in, 1 out]
            n657 = To Variant(anything=w1362) -> (Variant=w1366:variant)
            n658 = call <vilib>:"Q.Enqueue Task.vi"("Data1"=w1366, "Task Name"="Simulate", "Q In"=w1367) -> ()  [unwired: 7 in, 2 out]
          }
          frame "Show Block Diagram" {
            n659 = call <vilib>:"Module.Window, Q Task.vi"("Action"=Window.Task,_Action."Open Block Diagram()", "Q In"=w1369) -> ()  [unwired: 8 in, 2 out]
          }
          frame "Go to Maint Tab" {
            n660 = call <vilib>:"Module.Window, Q Task.vi"("Show"=TRUE, "Action"=Window.Task,_Action."Go To Maint Tab()", "Q In"=w1372) -> ()  [unwired: 7 in, 2 out]
          }
        }
      }
      event Panel Resize {
        n661 = event-data() -> ()  [unwired: 1 in, 8 out]
        n662 = case shown="True" FALSE {
          tunnel: w1374 -> [_ w1376]
          frame False {
          }
          frame True {
            n663 = call <vilib>:"Module.Window, Q Task.vi"("Action"=Window.Task,_Action."Resize()", "Q In"=w1376) -> ()  [unwired: 8 in, 2 out]
          }
        }
      }
      event "Set Window Bounds": Value Change {
        n664 = event-data() -> ()  [unwired: 1 in, 6 out]
        n665 = control-ref of="This VI"() -> (w1379:refnum<vi>)
        n666 = property class="VI"(reference=w1379, "Front Panel.WinBounds"="New Window Bounds", "Front Panel.Resizeable"=TRUE ("Front Panel Window:Resizable")) -> ("Front Panel.PanelBounds"=→"Old Window Bounds":T8)  [unwired: 1 in, 2 out]
      }
      event "Leave Maint": Value Change {
        n667 = event-data() -> ()  [unwired: 1 in, 6 out]
        n668 = local write "Main Tab"(0) -> ()
      }
      event Value Change {
        n669 = event-data() -> ()  [unwired: 1 in, 6 out]
        n670 = To Variant(anything="Logging Level") -> (Variant=w1383:variant)
        n671 = call <vilib>:"Q.Enqueue App.vi"("Data1"=w1383, "Task Name"="Set Logging Level", "Q In"=w1384) -> ()  [unwired: 7 in, 2 out]
      }
      event "Abort": Value Change {
        n672 = event-data() -> ()  [unwired: 1 in, 6 out]
        n673 = call <vilib>:"Scheduler.Clear-Reset.vi"("Q In"=w1388) -> ("error out"=w1390:errorcluster, "Q Out"=w1389:refnum<queue>)  [unwired: 9 in]
        n674 = Flush Queue(queue=w1389, error in (no error)=w1390) -> (queue out=w1387:refnum<queue>)  [unwired: 2 out]
        n675 = call <vilib>:"Q.Enqueue Task.vi"("Task Name"="Test Abort", "Q In"=w1387) -> ()  [unwired: 8 in, 2 out]
        n676 = for {
          N: 5 -> [_]
          n677 = call "Abort.Send Abort or Done Notificaiton.vi"("Abort(T)/Done(F)"=TRUE) -> ()  [unwired: 10 in, 1 out]
          n678 = Wait (ms)(milliseconds to wait=u32 10) -> ()  [unwired: 1 out]
        }
      }
      event "Test Reset": Value Change {
        n679 = event-data() -> ()  [unwired: 1 in, 6 out]
        n680 = call <vilib>:"Q.Enqueue Task.vi"("Task Name"="Test Reset", "Q In"=w1394) -> ()  [unwired: 8 in, 2 out]
      }
      event "Filter", "Show Only Failures": Value Change {
        n681 = event-data() -> ()  [unwired: 1 in, 6 out]
        n682 = call <vilib>:"Q.Enqueue Task.vi"("Task Name"="Update Results", "Q In"=w1396) -> ()  [unwired: 8 in, 2 out]
      }
      event "Get Top SN": Value Change {
        n683 = event-data() -> ()  [unwired: 1 in, 6 out]
        n684 = Build Array("GetUUTSN", "TopSN") -> (w1400:string[])
        n685 = To Variant(anything=w1400) -> (Variant=w1401:variant)
        n686 = call <vilib>:"Q.Enqueue Task.vi"("Data1"=w1401, "Task Name"="Funct Local Call", "Q In"=w1402) -> ()  [unwired: 7 in, 2 out]
      }
      event "Check UUT Enum Status": Value Change {
        n687 = event-data() -> ()  [unwired: 1 in, 6 out]
        n688 = Build Array("CheckUutEnumStatus") -> (w1405:string[])
        n689 = To Variant(anything=w1405) -> (Variant=w1406:variant)
        n690 = call <vilib>:"Q.Enqueue Task.vi"("Data1"=w1406, "Task Name"="Funct Local Call", "Q In"=w1407) -> ()  [unwired: 7 in, 2 out]
      }
      event "Run SoundCheck Script": Value Change {
        n691 = event-data() -> ()  [unwired: 1 in, 6 out]
        n692 = property on="Audio Seq Name" class="Ring (strict)"() -> ("RingText.Text"=w1409:string)  [unwired: 2 in, 2 out]
        n693 = Build Array("RunAudioScript", w1409) -> (w1411:string[])
        n694 = To Variant(anything=w1411) -> (Variant=w1412:variant)
        n695 = call <vilib>:"Q.Enqueue Task.vi"("Data1"=w1412, "Task Name"="Funct Local Call", "Q In"=w1413) -> ()  [unwired: 7 in, 2 out]
      }
      event "Run Audio Check": Value Change {
        n696 = event-data() -> ()  [unwired: 1 in, 6 out]
        n697 = Build Array("RunAudioCheckUtil") -> (w1416:string[])
        n698 = To Variant(anything=w1416) -> (Variant=w1417:variant)
        n699 = call <vilib>:"Q.Enqueue Task.vi"("Data1"=w1417, "Task Name"="Funct Local Call", "Q In"=w1418) -> ()  [unwired: 7 in, 2 out]
      }
      event "Init UUT Folder": Value Change {
        n700 = event-data() -> ()  [unwired: 1 in, 6 out]
        n701 = Build Array("Create_UUTFolder") -> (w1420:string[])
        n702 = To Variant(anything=w1420) -> (Variant=w1421:variant)
        n703 = call <vilib>:"Q.Enqueue Task.vi"("Data1"=w1421, "Task Name"="Funct Local Call", "Q In"=w1423) -> ()  [unwired: 7 in, 2 out]
      }
      event "Parse Results": Value Change {
        n704 = event-data() -> ()  [unwired: 1 in, 6 out]
        n705 = Build Array("ParseAudioResults") -> (w1425:string[])
        n706 = To Variant(anything=w1425) -> (Variant=w1426:variant)
        n707 = call <vilib>:"Q.Enqueue Task.vi"("Data1"=w1426, "Task Name"="Funct Local Call", "Q In"=w1428) -> ()  [unwired: 7 in, 2 out]
      }
      event "Parse Mic. Seal Results": Value Change {
        n708 = event-data() -> ()  [unwired: 1 in, 6 out]
        n709 = Build Array("ParseMicrophoneCoveredResults") -> (w1431:string[])
        n710 = To Variant(anything=w1431) -> (Variant=w1432:variant)
        n711 = call <vilib>:"Q.Enqueue Task.vi"("Data1"=w1432, "Task Name"="Funct Local Call", "Q In"=w1430) -> ()  [unwired: 7 in, 2 out]
      }
      event "Config - Reset": Value Change {
        n712 = event-data() -> ()  [unwired: 1 in, 6 out]
        n713 = call <vilib>:"Q.Enqueue Task.vi"("Task Name"="Config - Reset Audio Limit Config", "Q In"=w1436) -> ()  [unwired: 8 in, 2 out]
      }
      event "Archive Results": Value Change {
        n714 = event-data() -> ()  [unwired: 1 in, 6 out]
        n715 = call "File.Date String, File Safe.vi"() -> ("Date"=w1437:string)  [unwired: 3 in]
        n716 = Build Array("Archive_Results", "Mode", w1437) -> (w1440:string[])
        n717 = To Variant(anything=w1440) -> (Variant=w1441:variant)
        n718 = call <vilib>:"Q.Enqueue Task.vi"("Data1"=w1441, "Task Name"="Funct Local Call", "Q In"=w1442) -> ()  [unwired: 7 in, 2 out]
      }
      event "Open UUT Dir", "Open Summary Dir", "Open Archive Dir": Value Change {
        n719 = event-data() -> ()  [unwired: 1 in, 6 out]
        n720 = local read "Archive Summary Dir"() -> (w1448:path)
        n721 = local read "Archive Dir"() -> (w1449:path)
        n722 = local read "UUT Dir"() -> (w1450:path)
        n723 = case shown="False" "Open UUT Dir" {
          tunnel: w1450 -> [_ w1457]
          tunnel: w1449 -> [w1452 _]
          tunnel: w1448 -> [w1451 _]
          tunnel: [w1453 w1457] -> w1446
          tunnel: "Open Archive Dir" -> [w1454 _]
          frame False {
            n724 = case shown="True" w1454 {
              tunnel: [w1455 w1456] -> w1453
              tunnel: w1452 -> [_ w1456]
              tunnel: w1451 -> [w1455 _]
              frame False {
              }
              frame True {
              }
            }
          }
          frame True {
          }
        }
        n725 = call <vilib>:"File.Open File or Folder.vi"("Path"=w1446) -> ("Error Out"=w1445:errorcluster)  [unwired: 10 in]
        n726 = call <vilib>:"Clear Errors.vi"("error in (no error)"=w1445) -> ()  [unwired: 5 in, 2 out]
      }
      event "Clear Errors": Value Change {
        n727 = event-data() -> ()  [unwired: 1 in, 6 out]
        n728 = call "Error.Clear.vi"("Q In"=w1458) -> ()  [unwired: 9 in, 2 out]
      }
      event "SN": Value Change {
        n729 = event-data() -> ()  [unwired: 1 in, 6 out]
        n730 = To Variant(anything="SN") -> (Variant=w1459:variant)
        n731 = call <vilib>:"Q.Enqueue Task.vi"("Data1"=w1459, "Task Name"="Update SN", "Q In"=w1462) -> ()  [unwired: 7 in, 2 out]
      }
      event "Left Mic Cover": Value Change {
        n732 = event-data() -> ()  [unwired: 1 in, 6 out]
        n733 = case shown="False" "Left Mic Cover" {
          tunnel: ["0" "1"] -> w1467
          frame False {
          }
          frame True {
          }
        }
        n734 = Build Array(w1467, "Left" ("element"), "False" ("element"), "1" ("element")) -> (w1464:string[])
        n735 = To Variant(anything=w1464) -> (Variant=w1471:variant)
        n736 = call <vilib>:"Q.Enqueue Function.vi"("Q Name"="SERVO", "Data1"=w1471, "Task Name"="Move", "Q In"=w1470) -> ()  [unwired: 5 in, 3 out]
      }
      event "Right Mic Cover": Value Change {
        n737 = event-data() -> ()  [unwired: 1 in, 6 out]
        n738 = case shown="False" "Right Mic Cover" {
          tunnel: ["0" "1"] -> w1481
          frame False {
          }
          frame True {
          }
        }
        n739 = Build Array(w1481, "Right" ("element"), "False" ("element"), "1" ("element")) -> (w1478:string[])
        n740 = To Variant(anything=w1478) -> (Variant=w1483:variant)
        n741 = call <vilib>:"Q.Enqueue Function.vi"("Q Name"="SERVO", "Data1"=w1483, "Task Name"="Move", "Q In"=w1476) -> ()  [unwired: 5 in, 3 out]
      }
      event "Both Mics": Value Change {
        n742 = event-data() -> ()  [unwired: 1 in, 6 out]
        n743 = case shown="True" "Both Mics" {
          tunnel: ["0" "1"] -> w1494
          tunnel: [FALSE TRUE] -> w1487
          frame False {
          }
          frame True {
          }
        }
        n744 = property on="Right Mic Cover" class="Bool (strict)"("Value"=w1487) -> ()  [unwired: 2 in, 2 out]
        n745 = property on="Left Mic Cover" class="Bool (strict)"("Value"=w1487) -> ()  [unwired: 2 in, 2 out]
        n746 = Build Array(w1494, "All" ("element"), "False" ("element"), "1" ("element")) -> (w1491:string[])
        n747 = To Variant(anything=w1491) -> (Variant=w1496:variant)
        n748 = call <vilib>:"Q.Enqueue Function.vi"("Q Name"="SERVO", "Data1"=w1496, "Task Name"="Move", "Q In"=w1489) -> ()  [unwired: 5 in, 3 out]
      }
      event "UUT Dir": Value Change {
        n749 = event-data() -> ()  [unwired: 1 in, 6 out]
        n750 = To Variant(anything="UUT Dir") -> (Variant=w1503:variant)
        n751 = call <vilib>:"Q.Enqueue Task.vi"("Data1"=w1503, "Task Name"="Update UUT Folder", "Q In"=w1505) -> ()  [unwired: 7 in, 2 out]
      }
      event "Undock HMD Util", "Undock Servo Util": Value Change {
        n752 = event-data() -> ()  [unwired: 1 in, 6 out]
        n753 = Select(t="Module Undock - HMD" ("Task Name"), s="Undock HMD Util", f="Module Undock - Servo" ("Task Name")) -> (s? t:f=w1509:string)
        n754 = call <vilib>:"Q.Enqueue Task.vi"("Task Name"=w1509, "Q In"=w1510) -> ()  [unwired: 8 in, 2 out]
      }
      event Timeout {
        n755 = event-data() -> ()  [unwired: 1 in, 3 out]
        n756 = local read "Test Running"() -> (w1511:bool)
        n757 = case shown="False" w1511 {
          frame False {
          }
          frame True {
            n758 = local read "Start Time"() -> (w1512:timestamp)
            n759 = Get Date/Time In Seconds() -> (seconds since 1Jan1904=w1513:timestamp)
            n760 = Subtract(x=w1513, y=w1512) -> (x-y=w1514:dbl)
            n761 = local write "Duration(s)"(w1514) -> ()
          }
        }
      }
    }
  }
  "Title" <- w5
